vi "TV-HR_Main.vi"(8 "error in":errorcluster) -> (0 "error out":errorcluster)   [LabVIEW 2024]
uses:
  Buttons/Zoom IN.ctl
  Buttons/Zoom Out.ctl
  Buttons/Zoom Inn.ctl
  Buttons/Zoom Fit.ctl
  Buttons/ML Analysis.ctl
  <vilib>/Utility/error.llb/DialogType.ctl
  Controls/RVHR - UI Refs.ctl
  Controls/RVHR - Reporting Settings.ctl
  Controls/RVHR - Local Data.ctl
  Controls/Test Cluster.ctl
  Controls/Excluded Information.ctl
  Controls/Language.ctl
  Controls/Device_Type.ctl
  <vilib>/Utility/miscctls.llb/LVRectTypeDef.ctl
  <vilib>/Utility/miscctls.llb/LVBoundsTypeDef.ctl
  Modules/Error handling/Controls/Error Command.ctl
  Controls/DB FTR Commands.ctl
  <vilib>/Utility/miscctls.llb/LVPoint32TypeDef.ctl
  Controls/Print Command.ctl
  Controls/RVHR - Analysis Mode.ctl
  Controls/Run Listbox Command.ctl
panel:
  in  "Ref Profile":string caption="Ref Profile:"
  in  "Company":string caption="Company:"
  in  "Location":string caption="Location:"
  in  "Operator":string caption="Operator:"
  in  "Notes":string caption="Notes:"
  in  "Date":string caption="Date:"
  in  "Run End":dbl caption="Run End:" format="%.3f km"
  in  "Run Start":dbl caption="Run Start:" format="%.3f km"
  out "new picture":picture
  out "EN Sub-Title":string caption="EN13231-2/EN13231-3"
  out "Sub-Title":string caption="RV-HR Report"
  out "Title":string caption="Rail Vision - HR"
  out "ML Analysis":T1
  in  "All?":bool
  in  "Run Selection Listbox":i32(listbox)
  in  "Feature Type:":u16(ring) items=["Clip", "Crack", "Add New..."]
  in  "Run Distance":dbl(slide) caption="Distance (km)" min=11.015 max=11.025 step=0.002 scale=11.015..11.025
  out "Running?":bool
  in  "Zoom Toolbar L":T5
  out "Rail Preview":picture
  in  "Zoom Window":T6
  out "Image Preview":picture
  in  "Previous?":bool
  in  "Next?":bool
  out "Page":string
  out "Left Rail":string
  out "Image":picture
  # "Left"
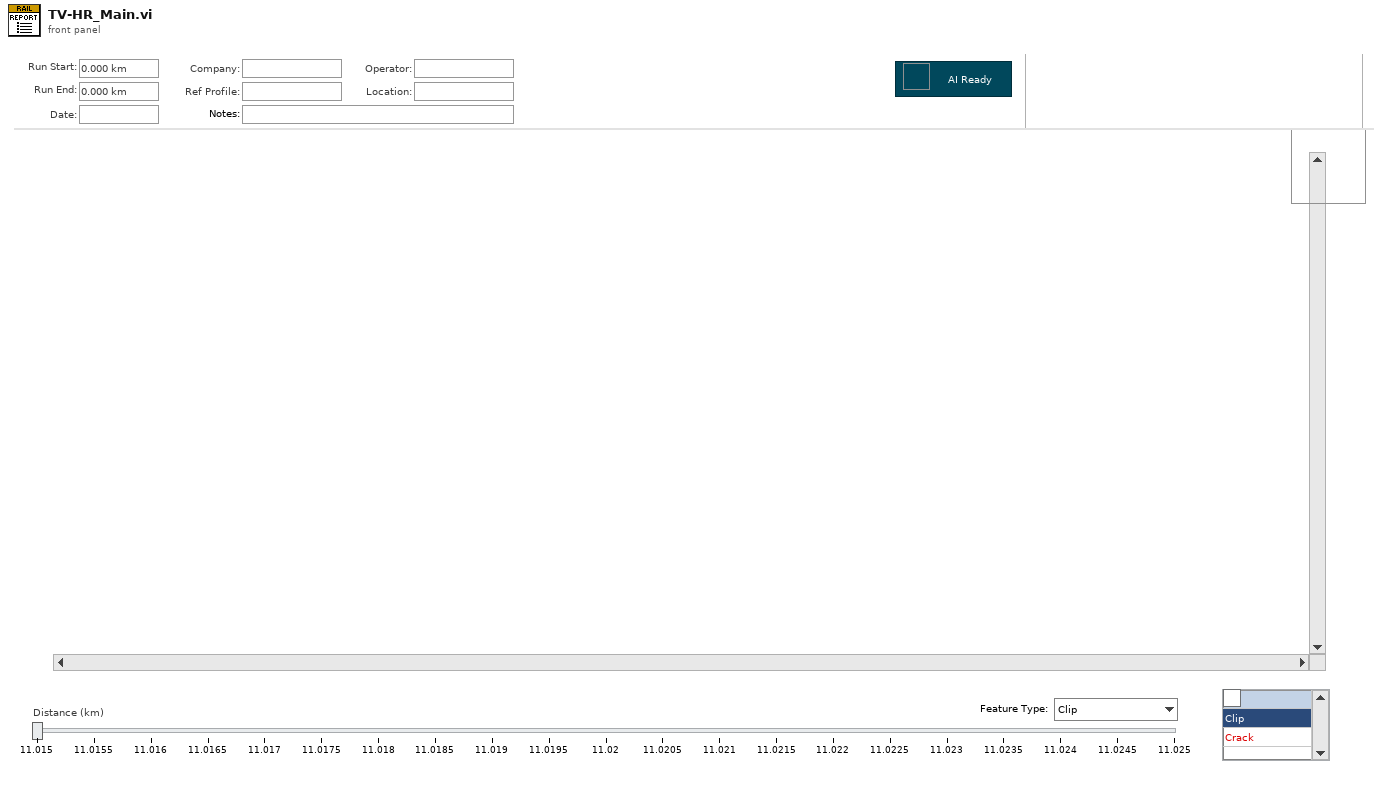
[diagram p1: front panel]
types:
  T1 = typedef "ML Analysis.ctl" = bool
  T2 = typedef "Zoom Out.ctl" = bool
  T3 = typedef "Zoom Inn.ctl" = bool
  T4 = typedef "Zoom Fit.ctl" = bool
  T5 = cluster{"Zoom Out":T2, "Zoom In":T3, "Zoom Fit":T4}
  T6 = typedef "Zoom IN.ctl" = bool
  T7 = typedef "DialogType.ctl" = u16
  T8 = typedef "RVHR - UI Refs.ctl" = cluster{"Title":refnum<vi>, "Sub-Title":refnum<vi>, "EN Sub-Title":refnum<vi>, "Run Start":refnum<vi>, "Run End":refnum<vi>, "Date":refnum<vi>, "Company":refnum<vi>, "Ref Profile":refnum<vi>, "Operator":refnum<vi>, "Location":refnum<vi>, "Notes":refnum<vi>, "Left Rail":refnum<vi>, "Page":refnum<vi>, "Image":refnum<vi>, "Run Distance":refnum<vi>, "Next?":refnum<vi>, "Previous?":refnum<vi>, "Image Preview":refnum<vi>, "Feature Type:":refnum<vi>, "Zoom Toolbar L":refnum<vi>, "Rail Preview":refnum<vi>, "ML Analysis":refnum<vi>, "Running?":refnum<vi>, "All?":refnum<vi>, "Run Selection Listbox":refnum<vi>}
  T9 = typedef "RVHR - Reporting Settings.ctl" = cluster{"Image Distance (m)":dbl}
  T10 = typedef "Error Command.ctl" = enum16{"Initialisation", "Handle", "Close"}
  T11 = enum8{"Enabled", "Disabled", "Disabled and Grayed Out"}
  T12 = typedef "RVHR - Analysis Mode.ctl" = enum16{"Current Images", "Full Run"}
  T13 = enum16{"Get Image", "Get Preview", "Add", "Remove"}
  T14 = cluster{"Label.Text":string, "Mouse Position (Start)":cluster{"X":i32, "Y":i32}}
  T15 = typedef "DB FTR Commands.ctl" = enum16{"Add New", "Get", "Update"}
  T16 = typedef "LVPoint32TypeDef.ctl" = cluster{"Horizontal":i32, "Vertical":i32}
  T17 = typedef "Print Command.ctl" = enum16{"Current Page", "Full Report"}
  T18 = typedef "Run Listbox Command.ctl" = enum16{"Init", "Item Names", "Update", "Update All", "Get Selections", "Clear"}
  T19 = typedef "Language.ctl" = enum16{"English", "Chinese", "German"}
  T20 = typedef "Supervisory Config Cluster.ctl" = cluster{"UI Information":T21, "Test Cluster":T25, "RV-HR Settings Cluster":T26}
  T21 = typedef "UI Init Config Info.ctl" = cluster{"Header Image":path, "Language":T19, "First Run?":bool, "Setup Camera?":bool, "Device Type":T22, "Encoder Type":T23, "Version":T24, "port":i32, "greyscale":bool, "camera index":i32}
  T22 = typedef "Device_Type.ctl" = enum16{"CAT", "Bi-CAT", "YRCA", "RCA", "RV-HR", "TV-HR"}
  T23 = typedef "EncoderType.ctl" = enum16{"Tacho", "Quadrature"}
  T24 = typedef "Software Version.ctl" = enum16{"RailMeasurement_CAT", "RailMeasurement_Master", "RailMeasurement_RCA", "RailMeasurement_CAT-V", "RailMeasurement_RCA-V", "RailMeasurement_RV-HR"}
  T25 = typedef "Test Cluster.ctl" = cluster{"Operator":string, "Description":string, "Line":string, "Start Position":dbl, "Run Length":dbl, "Sensor A Position":dbl, "Rail Side":bool, "Distance Direction":bool, "Path":path, "Sensor B Position":dbl, "Visible Chart Distance":dbl, "Company":string, "Ref Profile":string}
  T26 = typedef "Settings Cluster.ctl" = cluster{"Sensor A Calibration":dbl, "Integrator Time":dbl, "Encoder Spacing":dbl, "Encoder Threshold":dbl, "Sampling Distance":T27, "Swap Direction?":bool, "Min Walking Speed":dbl, "Max Walking Speed":dbl, "Distance Format":T28, "Sensor B Calibration":dbl, "Tacho Pulses/Rev":dbl, "Wheel Diameter":dbl, "Max Short Roughness":dbl, "Max Long Roughness":dbl, "Measuring Interval":dbl, "Measuring Length":dbl, "Wavelengths":dbl[], "Device Resolution":T29, "Detect Change in Direction?":bool, "Save Images?":bool, "Image Frequency":T27, "Save Video?":bool, "Image Offset":dbl, "Start Position at 0m?":bool, "Live Corrug Est.?":bool, "Wavelength Corrug":u8, "Distance Corrug":u8, "Update Corrug":u8}
  T27 = typedef "Sampling DIstance.ctl" = u16
  T28 = typedef "Distance Units.ctl" = u16
  T29 = typedef "Device_Resolution.ctl" = u16
  T30 = typedef "RVHR - Local Data.ctl" = cluster{"Main Filtered Data":dbl[][][], "Main Dist Data":dbl[], "Comp Filtered Data":dbl[][][], "Comp Dist Data":dbl[], "Image":u16, "Total Images":u16, "Main Test Cluster":T25, "Main Dates-Times":cluster{"Start Date":string, "Start Time":string, "Finish Time":string}, "Comp Test Cluster":T25, "Comp Dates-Times":cluster{"Start Date":string, "Start Time":string, "Finish Time":string}, "Comp Offset (mm)":i64, "XY Highlight Distance":dbl[], "Left Exc Info":T31[], "Right Exc Info":T31[], "Custom Start-Point":dbl, "UI Start-Distance":dbl, "UI End-Distance":dbl, "Distance Format":u8, "Language":T19, "Vision?":bool, "Left Image Folder":path, "Filename _L":string[], "Image Distances _L":dbl[], "Image Inc (km)":dbl, "Device Type":T22, "Panel Bounds":T32, "Panel Size":T33, "Version":string, "db Filepath":path, "Image Display Scale Factor":dbl}
  T31 = typedef "Excluded Information.ctl" = cluster{"Start Dist":dbl, "End Dist":dbl, "Comments":string}
  T32 = typedef "LVRectTypeDef.ctl" = cluster{"Left":i16, "Top":i16, "Right":i16, "Bottom":i16}
  T33 = typedef "LVBoundsTypeDef.ctl" = cluster{"Width":u32, "Height":u32}
  T34 = typedef "Language Vision Text Cluster.ctl" = cluster{"Home":string, "Test Setup":string, "Run Test":string, "Configure":string, "Hardware Viewer":string, "Review Test":string, "Report":string, "Exit":string, "Device Connected?":string, "Test in Progress?":string, "Simulate?":string, "Device Type 1":string, "Device Type 2":string, "Device Type 3":string, "Device Type 4":string, "Device Type 5":string, "Device Type 6":string, "Device Type 7":string, "Software Version":string, "Support":string, "Operator":string, "Test Description":string, "Line":string, "Test Folder Path":string, "Test Folder Path RCA":string, "Start Position":string, "Sensor Position":string, "Sensor A Position":string, "Sensor B Position":string, "Visible Chart Distance":string, "Rail Side":string, "Rail A Side":string, "Distance Direction":string, "Start":string, "Distance Travelled":string, "Current Position":string, "Stop Test":string, "Pause Test":string, "Displacement":string, "Position":string, "Sensor Calibration":string, "Sensor A Calibration":string, "Sensor B Calibration":string, "Encoder Spacing":string, "Sampling Distance":string, "Tacho Pulses/Rev":string, "Wheel Diameter":string, "Sampling Distances":string[], "Distance Unit":string, "Distance Units":string[], "Swap Direction":string, "Language":string, "Device Resolution":string, "Device Resolutions":string[], "Detect Change in Direction":string, "Save Config":string, "Encoder Data":string, "Sensor Data":string, "Sensor A Data":string, "Sensor B Data":string, "Voltage":string, "Time (m:s)":string, "Unit mm/s/V":string, "Unit mm":string, "Unit km":string, "Unit m":string, "Start Test Message":string, "Stop Test Message":string, "Exit Message":string, "File Exists Message":string, "File Path Invalid Message":string, "Combine Error":string, "Combine Success":string, "Roller Comp Error":string, "Test Folder Path (Live)":string, "Folder Error":string, "Enc Count":string, "Run Start":string, "Run End":string, "Date":string, "Train":string, "Location":string, "Notes":string, "Heading_1":string, "Heading_2":string, "Left Rail":string, "Right Rail":string, "Left Exclusions":string, "Right Exclusions":string, "Settings":string, "Wavelength Ranges":string, "Y-Axis Limits":string, "Exc Limits":string, "Other Settings":string, "Distance/Page":string, "Distance/Pages":string[], "Gridlines":string, "Report Tolerance":string, "Manual Cut":string, "Plot Colour":string, "Plot Colours":string[], "EN Standard":string, "RiL Standard":string, "Custom Standard":string, "Resolution":string, "Resolutions":string[], "Exceedence Header":string, "Distance (km)":string, "Left (%)":string, "Right (%)":string, "Page":string, "Align":string, "Main":string, "Comparison":string, "Offset":string, "From":string, "To":string, "Of":string, "File":string, "Load New":string, "Load Comparison":string, "Discard Comparison":string, "Print Current Page":string, "Print All Pages":string, "Print Exceedence Report":string, "Plot Main":string, "No Comparison Data to Align":string, "Run Load Error":string, "Report Load Error":string, "Cut":string, "Remove":string, "Config Settings Unsaved":string, "Acquisition Paused":string, "Please Select One Option Below":string, "RCA is Now Stationary":string, "Reporting Setting":string, "Main Abbreviated":string, "Comparison Abbreviated":string, "Exceedence Abbreviated":string, "Align Comparison":string, "Rail Corrugation Analyser Reporting":string, "Show Exc. % in Graph":string, "Evaluate Sections <100m":string, "Evaluate Sections <0.062mile":string, "Section Too Short for Evaluation":string, "Language Change Prompt":string, "Show All":string, "Sections_km":string, "Sections_mi":string, "Vision":string, "Vision Report":string, "Vision Display":string, "Vision Displays":string[], "Save Images":string, "Image Frequency":string, "Section":string, "Brightness":string, "Contrast":string, "Shadow":string, "Sharpened":string, "Apply to all Images":string, "Reset":string, "Are you sure":string, "Image Processing":string, "Save Video":string, "Image Offset":string, "Camera Mode":string, "Camera Modes":string[], "Copy Page":string, "Copy Graphs":string, "Camera Mode Change Prompt":string, "Camera_1 Missing":string, "Camera_2 Missing":string, "Cameras Missing":string, "Camera Setup":string, "Camera_1 Connection Error":string, "Camera_2 Connection Error":string, "Cameras Connection Error":string, "No GPS":string, "No Signal":string, "Camera_1 Connected":string, "Camera_1 Not Connected":string, "Camera_2 Connected":string, "Camera_2 Not Connected":string, "Start Position at 0m?":string, "Continue":string, "New Test, Same Direction":string, "New Test, Opposite Direction":string, "Stop and Save":string, "Live Corrug Estimate":string, "Wavelength Corrug":string, "Distance Corrug ":string, "Update Corrug":string, "Company":string, "Ref Profile ":string, "Company_Report":string, "Ref Profile_Report":string, "Heading_1_RVHR":string, "Heading_2_RVHR":string, "Remove Feature":string, "Feature Type":string, "Feature Types":string[], "AI Not Ready":string}
  T35 = typedef "Vision - Local Data.ctl" = cluster{"Main Filtered Data":dbl[][][], "Main Dist Data":dbl[], "Comp Filtered Data":dbl[][][], "Comp Dist Data":dbl[], "Page":u8, "Total Pages":u8, "Main Test Cluster":T25, "Main Dates-Times":cluster{"Start Date":string, "Start Time":string, "Finish Time":string}, "Comp Test Cluster":T25, "Comp Dates-Times":cluster{"Start Date":string, "Start Time":string, "Finish Time":string}, "Comp Offset (mm)":i64, "XY Highlight Distance":dbl[], "Left Exc Info":T31[], "Right Exc Info":T31[], "Custom Start-Point":dbl, "UI Start-Distance":dbl, "UI End-Distance":dbl, "Distance Format":u8, "Language":T19, "Vision?":bool, "Image Folder":path, "Filename _L":string[], "Filename _R":string[], "Image Distances _L":dbl[], "Image Distances _R":dbl[], "Image Inc (km)":dbl, "Device Type":T22, "Panel Bounds":T32, "Panel Size":T33, "Vision Settings":T36}
  T36 = typedef "Vision - Reporting Settings.ctl" = cluster{"Show All?":bool, "Dist/Page":T37, "Sections":T38[]}
  T37 = typedef "Vision - Dist Per Page.ctl" = u16
  T38 = typedef "Vision - Section.ctl" = cluster{"From":dbl, "To":dbl, "Discard":T39}
  T39 = typedef "Bin.ctl" = bool
  T40 = typedef "imagedata.ctl" = cluster{"image type":i32, "image depth":i32, "image":u8[], "mask":u8[], "colors":u32[], "Rectangle":cluster{"left":i16, "top":i16, "right":i16, "bottom":i16}}
  T41 = typedef "Local Data.ctl" = cluster{"Main Filtered Data":dbl[][][], "Main Dist Data":dbl[], "Comp Filtered Data":dbl[][][], "Comp Dist Data":dbl[], "Page":u8, "Total Pages":u8, "Main Test Cluster":T25, "Main Dates-Times":cluster{"Start Date":string, "Start Time":string, "Finish Time":string}, "Comp Test Cluster":T25, "Comp Dates-Times":cluster{"Start Date":string, "Start Time":string, "Finish Time":string}, "Comp Offset (mm)":i64, "XY Highlight Distance":dbl[], "Left Exc Info":T31[], "Right Exc Info":T31[], "Custom Start-Point":dbl, "UI Start-Distance":dbl, "UI End-Distance":dbl, "Distance Format":u8, "Language":T19, "Main Sampling Distance (mm)":dbl, "Comp Sampling Distance (mm)":dbl}
  T42 = typedef "eventvkey.ctl" = enum16{"ASCII", "Enter", "Return", "Shift", "Ctrl", "Alt", "Cmd", "Opt", "Caps", "NumLock", "Clear", "Break", "Up", "Down", "Left", "Right", "Insert", "Delete", "Home", "End", "PageUp", "PageDown", "Escape", "Help", "Pause", "ScrollLock", "F1", "F2", "F3", "F4", "F5", "F6", "F7", "F8", "F9", "F10", "F11", "F12", "F13", "F14", "F15", "F16", "F17", "F18", "F19", "F20", "F21", "F22", "F23", "F24", "Play", "VolumeUp", "VolumeDown", "Mute", "Two Byte Char"}
  T43 = typedef "LVMouseTypeDef.ctl" = cluster{"Mouse Position":cluster{"X":i32, "Y":i32}, "Mouse Modifiers":cluster{"Button Down":bool, "Shift Mod":bool, "Menu Mod":bool, "Option Mod":bool}}
  T44 = cluster{"Label.Text":string, "Mouse Position":cluster{"X":i32, "Y":i32}}
  T45 = enum32{"invalid app kind", "Development System", "Run Time System", "Student Edition", "Embedded LabVIEW", "Evaluation", "Custom"}
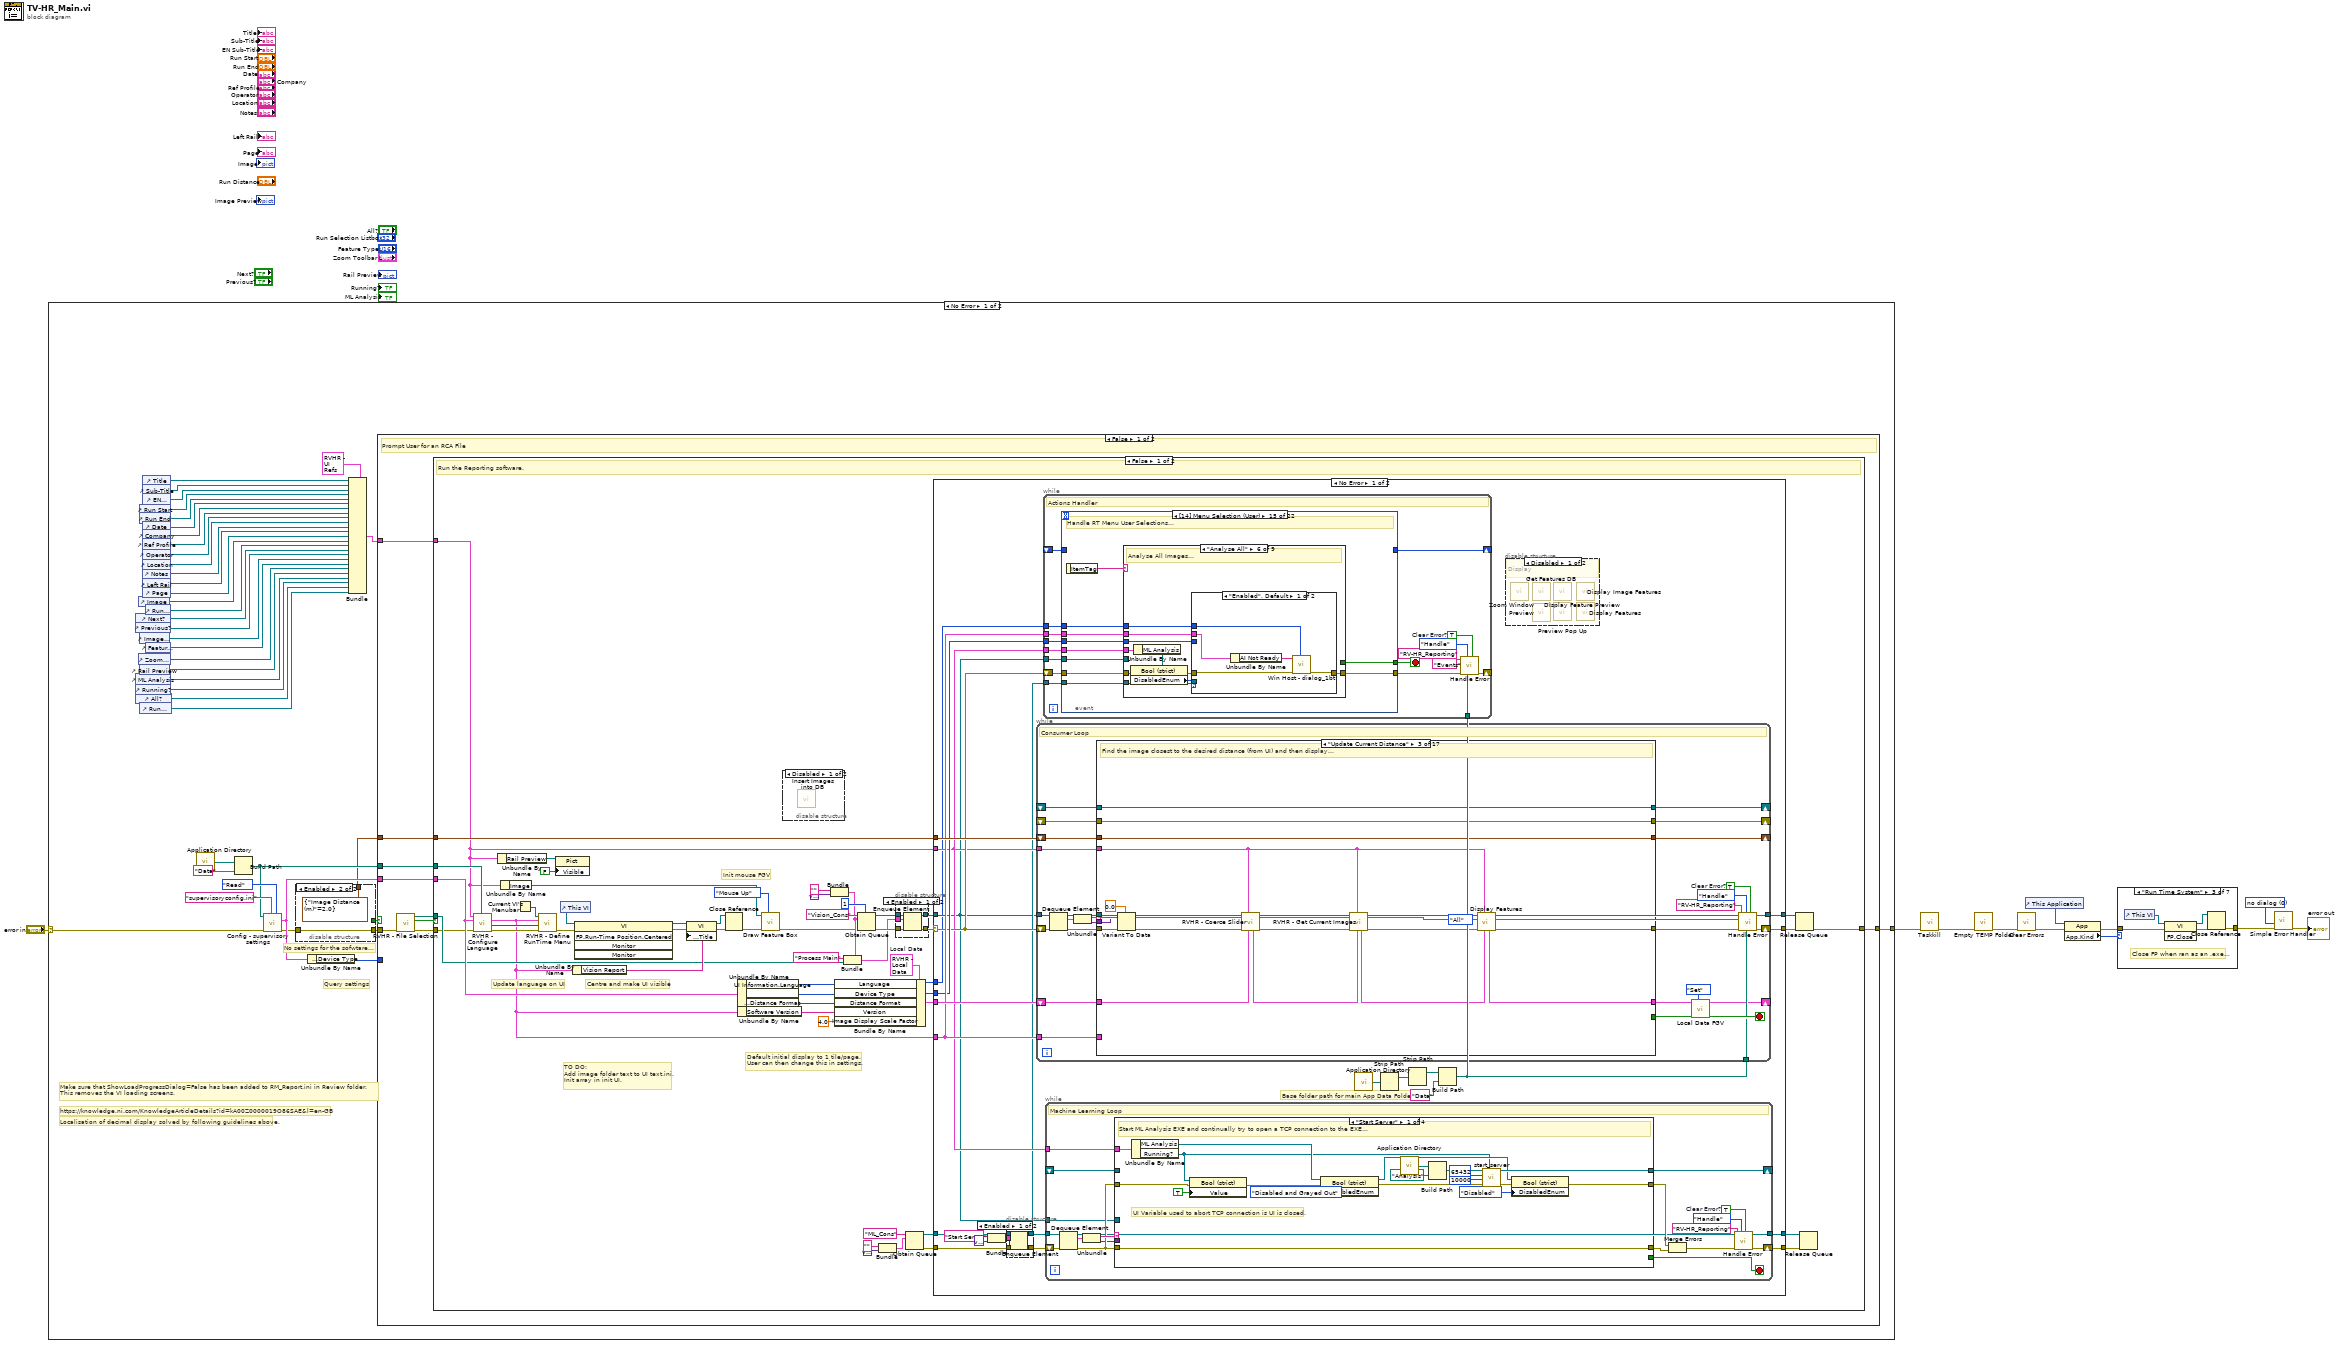
[diagram p0: block diagram]
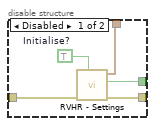
[diagram p2: hidden frame]
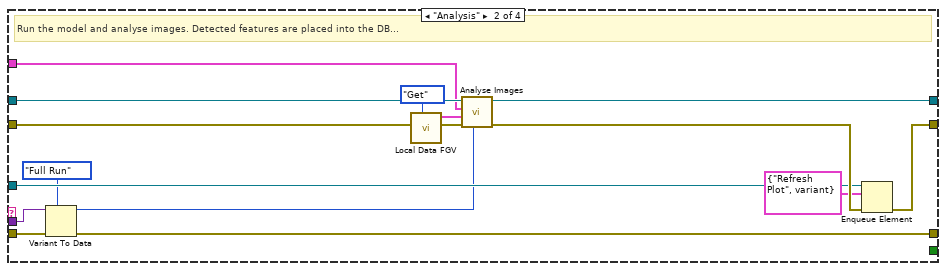
[diagram p6: hidden frame]
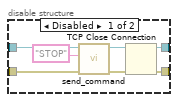
[diagram p8: hidden frame]
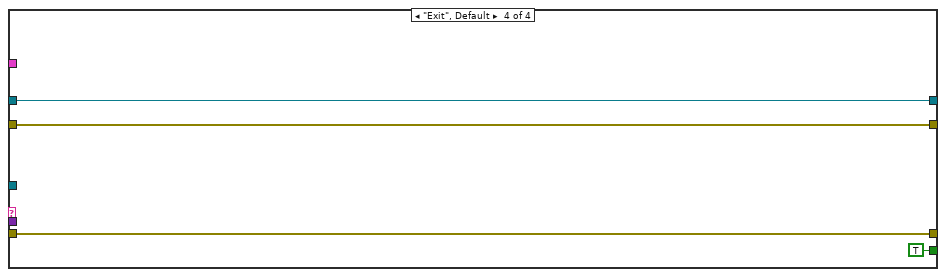
[diagram p9: hidden frame]
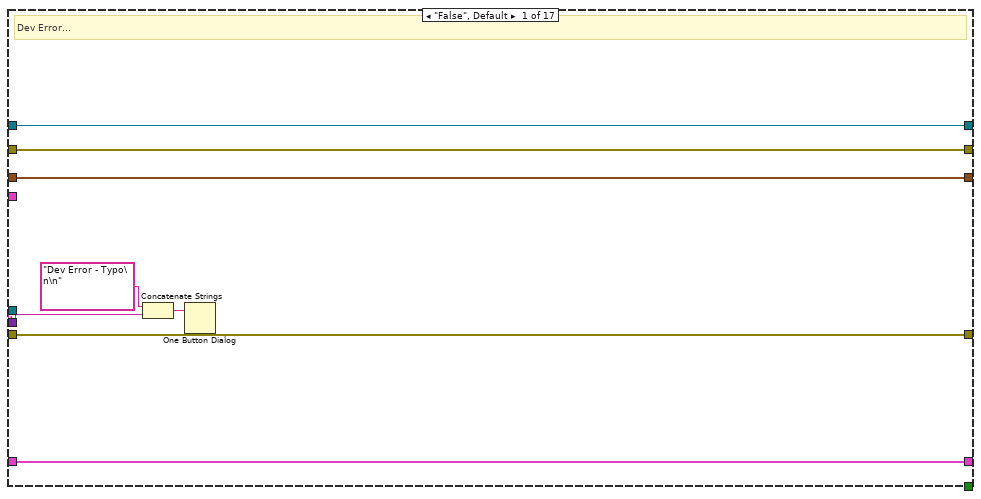
[diagram p11: hidden frame]
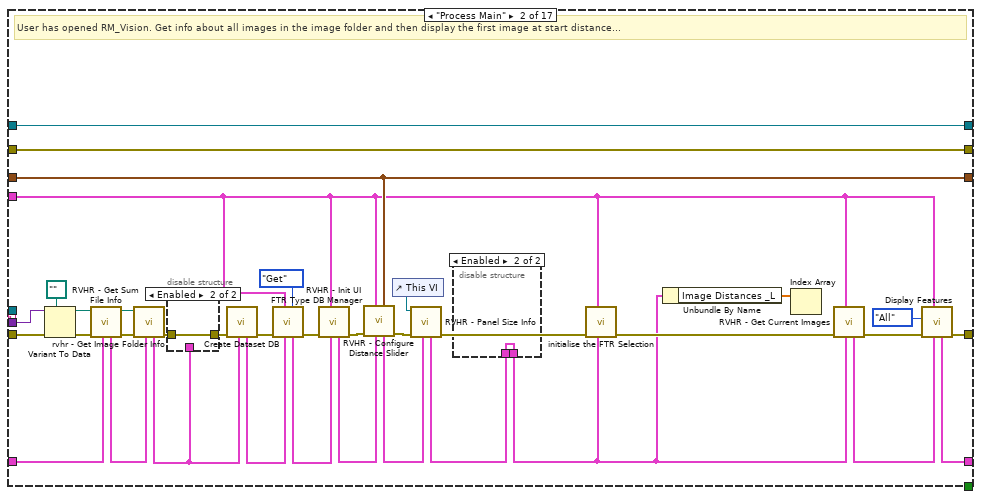
[diagram p12: hidden frame]
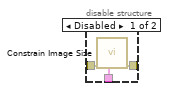
[diagram p13: hidden frame]
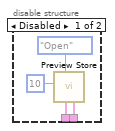
[diagram p14: hidden frame]
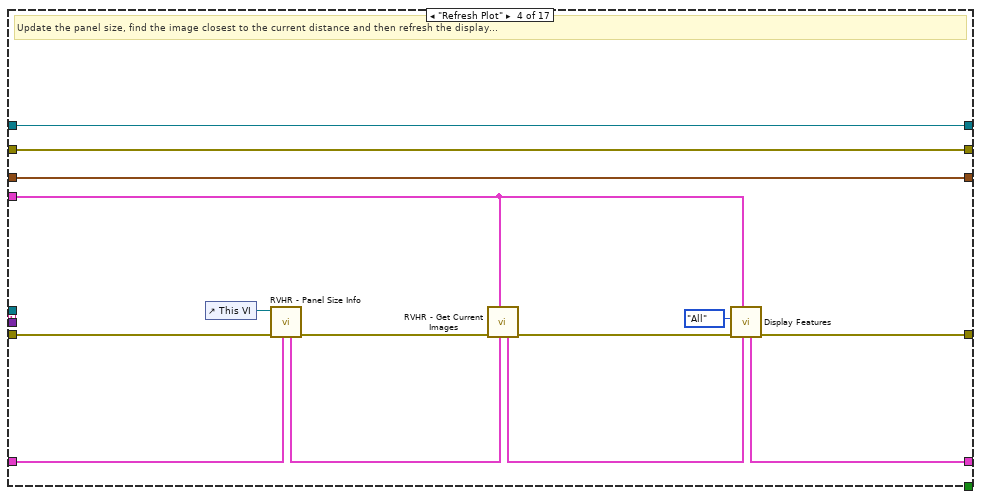
[diagram p15: hidden frame]
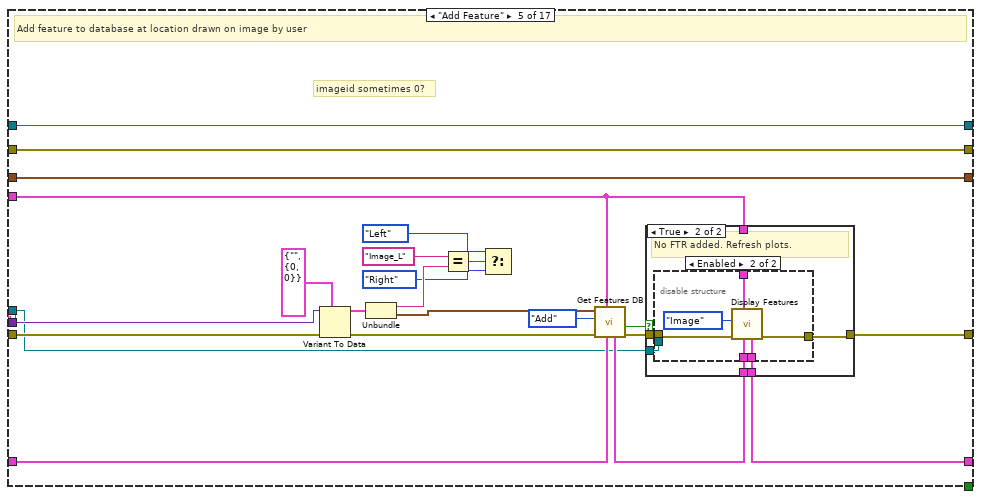
[diagram p16: hidden frame]
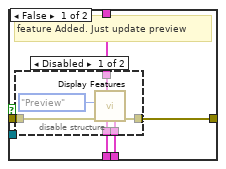
[diagram p17: hidden frame]
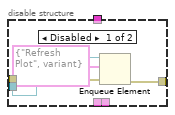
[diagram p19: hidden frame]
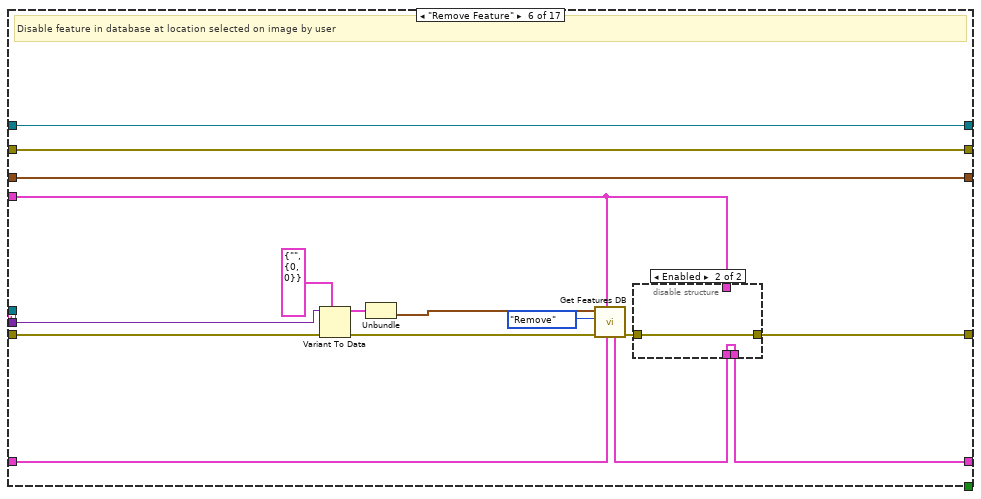
[diagram p20: hidden frame]
diagram:
  w8 = T7 0 items=["no dialog", "OK message", "continue or stop message", "OK message + warnings", "continue/stop + warnings"] ("type of dialog (OK msg:1)")
  n1 = case shown="No Error" "error in" {
    selector: "error in" -> [w18 w1098]
    tunnel: [w42 w1098] -> w5
    frame No Error {
      # "No settings for the sofwtare..."
      # "Make sure that ShowLoadProgressDialog=False has been added to RM_Report.ini in Review folder.\nThis removes the VI loading screens."
      # "Localisation of decimal display solved by following guidelines above."
      # "https://knowledge.ni.com/KnowledgeArticleDetails?id=kA00Z0000019O86SAE&l=en-GB"
      # "Query settings"
      n2 = control-ref of="Next?"() -> (w39:refnum<vi>)
      n3 = control-ref of="Previous?"() -> (w38:refnum<vi>)
      n4 = control-ref of="ML Analysis"() -> (w17:refnum<vi>)
      n5 = control-ref of="Running?"() -> (w16:refnum<vi>)
      n6 = control-ref of="All?"() -> (w14:refnum<vi>)
      n7 = control-ref of="Image"() -> (w19:refnum<vi>)
      n8 = control-ref of="Zoom Toolbar L"() -> (w20:refnum<vi>)
      n9 = control-ref of="Image Preview"() -> (w23:refnum<vi>)
      n10 = control-ref of="Rail Preview"() -> (w21:refnum<vi>)
      n11 = control-ref of="Run Selection Listbox"() -> (w13:refnum<vi>)
      n12 = control-ref of="Run Start"() -> (w31:refnum<vi>)
      n13 = control-ref of="Run End"() -> (w30:refnum<vi>)
      n14 = control-ref of="Title"() -> (w51:refnum<vi>)
      n15 = control-ref of="Sub-Title"() -> (w50:refnum<vi>)
      n16 = control-ref of="EN Sub-Title"() -> (w41:refnum<vi>)
      n17 = control-ref of="Date"() -> (w29:refnum<vi>)
      n18 = control-ref of="Company"() -> (w28:refnum<vi>)
      n19 = control-ref of="Ref Profile"() -> (w27:refnum<vi>)
      n20 = control-ref of="Operator"() -> (w26:refnum<vi>)
      n21 = control-ref of="Location"() -> (w25:refnum<vi>)
      n22 = control-ref of="Notes"() -> (w24:refnum<vi>)
      n23 = control-ref of="Left Rail"() -> (w49:refnum<vi>)
      n24 = control-ref of="Page"() -> (w44:refnum<vi>)
      n25 = control-ref of="Run Distance"() -> (w40:refnum<vi>)
      n26 = control-ref of="Feature Type:"() -> (w22:refnum<vi>)
      n27 = call <vilib>:"Application Directory.vi"() -> ("Application Directory"=w15:path)
      n28 = Build Path(base path=w15, name or relative path="Data") -> (appended path=w36:path)
      n29 = call "Config - supervisory settings.vi"(".ini Controller"=enum16{"Read", "Write"}."Read", ".ini filename"="supervisoryconfig.ini", "error in (no error)"=w18, "Directory Path"=w36) -> ("error out"=w32:errorcluster, "Supervisory Config Cluster Out"=w45:T20)  [unwired: 5 in, 1 out]
      n30 = disable-structure shown="Enabled" {
        disable-tunnel: [w56 T9 {"Image Distance (m)"=2.0} ("Supervisory Config Cluster In")] -> w35
        disable-tunnel: [w55 w58] -> w34
        disable-tunnel: [w54 _] -> w33
        disable-tunnel: w32 -> [w52 w58]
        frame Disabled {
          w53 = TRUE  # Initialise?
          n31 = call "RVHR - Settings.vi"("Initialise?"=w53, "error in (no error)"=w52) -> ("Error"=w55:errorcluster, "Cancelled?"=w54:bool, "Supervisory Config Cluster In"=w56:T9)  [unwired: 7 in]
        }
        frame Enabled {
        }
      }
      n32 = Unbundle By Name(w45) -> ("UI Information.Device Type"=w46:T22)
      n33 = Bundle(cluster=T8 {"Title"=refnum, "Sub-Title"=refnum, "EN Sub-Title"=refnum, "Run Start"=refnum, "Run End"=refnum, "Date"=refnum, "Company"=refnum, "Ref Profile"=refnum, "Operator"=refnum, "Location"=refnum, "Notes"=refnum, "Left Rail"=refnum, "Page"=refnum, "Image"=refnum, "Run Distance"=refnum, "Next?"=refnum, "Previous?"=refnum, "Image Preview"=refnum, "Feature Type:"=refnum, "Zoom Toolbar L"=refnum, "Rail Preview"=refnum, "ML Analysis"=refnum, "Running?"=refnum, "All?"=refnum, "Run Selection Listbox"=refnum} ("output cluster"), "Title"=w51, "Sub-Title"=w50, "EN Sub-Title"=w41, "Run Start"=w31, "Run End"=w30, "Date"=w29, "Company"=w28, "Ref Profile"=w27, "Operator"=w26, "Location"=w25, "Notes"=w24, "Left Rail"=w49, "Page"=w44, "Image"=w19, "Run Distance"=w40, "Next?"=w39, "Previous?"=w38, "Image Preview"=w23, "Feature Type:"=w22, "Zoom Toolbar L"=w20, "Rail Preview"=w21, "ML Analysis"=w17, "Running?"=w16, "All?"=w14, "Run Selection Listbox"=w13) -> (w43:T8)
      n34 = case shown="False" w33 {
        tunnel: w36 -> [w67 _]
        tunnel: w34 -> [w62 w1096]
        tunnel: w46 -> [_ _]
        tunnel: w45 -> [w66 _]
        tunnel: w43 -> [w65 _]
        tunnel: w35 -> [w64 _]
        tunnel: [w63 w1096] -> w42
        frame False {
          # "Prompt User for an RCA File"
          n35 = call "RVHR - File Selection.vi"("error in"=w62) -> ("error out"=w61:errorcluster, "cancelled?"=w60:bool, "RVHR path"=w59:path)  [unwired: 8 in]
          n36 = case shown="False" w60 {
            tunnel: w61 -> [w82 w1095]
            tunnel: w59 -> [w89 _]
            tunnel: w65 -> [w73 _]
            tunnel: w67 -> [w119 _]
            tunnel: w66 -> [w91 _]
            tunnel: w64 -> [w102 _]
            tunnel: [w104 w1094] -> w63
            frame False {
              w105 = T30 {"Main Filtered Data"=[[[0.0]]], "Main Dist Data"=[], "Comp Filtered Data"=[[[0.0]]], "Comp Dist Data"=[], "Image"=0, "Total Images"=0, "Main Test Cluster"={"Operator"="", "Description"="", "Line"="", "Start Position"=0.0, "Run Length"=0.0, "Sensor A Position"=0.0, "Rail Side"=FALSE, "Distance Direction"=FALSE, "Path"=path "", "Sensor B Position"=0.0, "Visible Chart Distance"=0.0, "Company"="", "Ref Profile"=""}, "Main Dates-Times"={"Start Date"="", "Start Time"="", "Finish Time"=""}, "Comp Test Cluster"={"Operator"="", "Description"="", "Line"="", "Start Position"=0.0, "Run Length"=0.0, "Sensor A Position"=0.0, "Rail Side"=FALSE, "Distance Direction"=FALSE, "Path"=path "", "Sensor B Position"=0.0, "Visible Chart Distance"=0.0, "Company"="", "Ref Profile"=""}, "Comp Dates-Times"={"Start Date"="", "Start Time"="", "Finish Time"=""}, "Comp Offset (mm)"=0, "XY Highlight Distance"=[], "Left Exc Info"=[], "Right Exc Info"=[], "Custom Start-Point"=0.0, "UI Start-Distance"=0.0, "UI End-Distance"=0.0, "Distance Format"=0, "Language"=enum."English", "Vision?"=FALSE, "Left Image Folder"=path "", "Filename _L"=[], "Image Distances _L"=[], "Image Inc (km)"=0.0, "Device Type"=enum."CAT", "Panel Bounds"={"Left"=0, "Top"=0, "Right"=0, "Bottom"=0}, "Panel Size"={"Width"=0, "Height"=0}, "Version"="", "db Filepath"=path "", "Image Display Scale Factor"=0.0}  # Local Data
              # "Init mouse FGV"
              # "Default initial display to 1 tile/page.\nUser can then change this in settings."
              # "TO DO:\nAdd image folder text to UI text.ini.\nInit array in init UI."
              # "Update language on UI"
              # "Centre and make UI visible"
              # "Run the Reporting software."
              n37 = call "RVHR - Configure Language.vi"("Directory Path"=w119, "error in (no error)"=w82, "Supervisory Config Cluster Out"=w91, "UI References"=w73) -> ("error out"=w101:errorcluster, "UI Information.Language"=w99:T19, "Language Config Cluster Out"=w70:T34)  [unwired: 4 in, 1 out]
              n38 = Unbundle By Name(w73) -> ("Rail Preview"=w86:refnum<vi>)
              n39 = Unbundle By Name(w73) -> ("Image"=w72:refnum<vi>)
              n40 = Current VI's Menubar() -> (w100:refnum<k9>)
              n41 = call "RVHR - Define RunTime Menu.vi"("error in (no error)"=w101, "Language"=w99, "Language Config Cluster Out"=w70, "Menu in"=w100) -> ("error out"=w98:errorcluster)  [unwired: 7 in]
              n42 = property class="Pict"(reference=w86, "Visible"=FALSE) -> ()  [unwired: 1 in, 2 out]
              n43 = control-ref of="This VI"() -> (w118:refnum<vi>)
              n44 = Unbundle By Name(w70) -> ("Vision Report"=w93:string)
              n45 = invoke class="VI" method="FP.Run-Time Position.Centered"(reference=w118, error in=w98) -> (reference out=w94:refnum<vi>, error out=w95:errorcluster)  [unwired: 3 in, 3 out]
              n46 = property class="VI"(reference=w94, error in=w95, "Front Panel.Title"=w93) -> (reference out=w97:refnum<vi>, error out=w96:errorcluster)
              n47 = Close Reference(reference=w97, error in (no error)=w96) -> (error out=w84:errorcluster)
              n48 = Unbundle By Name(w91) -> ("UI Information.Language"=w69:T19, "UI Information.Device Type"=w90:T22, "RV-HR Settings Cluster.Distance Format"=w92:T28)
              n49 = Unbundle By Name(w70) -> ("Software Version"=w71:string)
              n50 = call "Draw Feature Box.vi"("Action"=enum16{"Mouse Move", "Mouse Down", "Mouse Up"}."Mouse Up", "error in (no error)"=w84, "CtlRef"=w72) -> ("error out"=w83:errorcluster)  [unwired: 6 in, 2 out]
              n51 = disable-structure shown="Disabled" {
                frame Disabled {
                  n52 = call "Insert Images into DB.vi"() -> ()  [unwired: 12 in]
                }
                frame Enabled {
                }
              }
              n53 = Bundle("Command"="", "Data"=variant) -> (w113:cluster{"Command":string, "Data":variant})  [unwired: 1 in]
              n54 = Bundle By Name(cluster=w105, "Language"=w69, "Device Type"=w90, "Distance Format"=w92, "Version"=w71, "Image Display Scale Factor"=4.0) -> (w103:T30)
              n55 = Bundle(cluster=w113, "Command"="Process Main", "Data"=w89) -> (w111:cluster{"Command":string, "Data":variant})
              n56 = Obtain Queue(max queue size (-1, unlimited)=1, name (unnamed)="Vision_Cons", element data type=w113, error in (no error)=w83) -> (queue out=w110:refnum<queue>, error out=w115:errorcluster)  [unwired: 1 in, 1 out]
              n57 = Bundle("Command"="", "Data"=variant) -> (w80:cluster{"Command":string, "Data":variant})  [unwired: 1 in]
              n58 = disable-structure shown="Enabled" {
                disable-tunnel: w115 -> [w124 w125]
                disable-tunnel: w111 -> [w123 _]
                disable-tunnel: w110 -> [w122 w126]
                disable-tunnel: [w121 w126] -> w109
                disable-tunnel: [w120 w125] -> w85
                frame Enabled {
                  n59 = Enqueue Element(queue=w122, element=w123, error in (no error)=w124) -> (queue out=w121:refnum<queue>, error out=w120:errorcluster)  [unwired: 1 in, 1 out]
                }
                frame Disabled {
                }
              }
              n60 = Obtain Queue(name (unnamed)="ML_Cons", element data type=w80) -> (queue out=w77:refnum<queue>, error out=w76:errorcluster)  [unwired: 3 in, 1 out]
              n61 = case shown="No Error" w85 {
                selector: w85 -> [w140 w1090]
                tunnel: w109 -> [w128 w1091]
                tunnel: [w150 w1091] -> w108
                tunnel: [w149 errorcluster {"status"=FALSE, "code"=0, "source"=""} ("error IO")] -> w107
                tunnel: w102 -> [w148 _]
                tunnel: w73 -> [w139 _]
                tunnel: w103 -> [w147 w1085]
                tunnel: w70 -> [w142 w1087]
                tunnel: w90 -> [w141 _]
                tunnel: w77 -> [w130 w1083]
                tunnel: w76 -> [w132 w1082]
                tunnel: [w137 w1082] -> w75
                tunnel: [w136 w1083] -> w74
                tunnel: w69 -> [w127 _]
                frame No Error {
                  # "Base folder path for main App Data Folder"
                  n62 = Bundle("Command"="Start Server", "Data"=variant) -> (w133:cluster{"Command":string, "Data":variant})  [unwired: 1 in]
                  n63 = disable-structure shown="Enabled" {
                    disable-tunnel: w133 -> [w155 _]
                    disable-tunnel: w132 -> [w154 w156]
                    disable-tunnel: [w153 w156] -> w131
                    disable-tunnel: w130 -> [w152 w157]
                    disable-tunnel: [w151 w157] -> w129
                    frame Enabled {
                      n64 = Enqueue Element(queue=w152, element=w155, error in (no error)=w154) -> (queue out=w151:refnum<queue>, error out=w153:errorcluster)  [unwired: 1 in, 1 out]
                    }
                    frame Disabled {
                    }
                  }
                  n65 = while {
                    shift-right: [w174] -> _
                    shift-left: _ -> [w173]
                    tunnel: w139 -> [w172]
                    tunnel: w129 -> [w171]
                    shift-right: [w162] -> w137
                    shift-left: w131 -> [w170]
                    tunnel: [w161] -> w136
                    tunnel: w128 -> [w159]
                    stop <- w160 stop-if-true
                    w166 = TRUE  # Clear Error?
                    # "Machine Learning Loop"
                    n66 = Dequeue Element(queue=w171, error in (no error)=w170) -> (queue out=w161:refnum<queue>, element=w176:cluster{"Command":string, "Data":variant}, error out=w167:errorcluster)  [unwired: 1 in, 1 out]
                    n67 = Unbundle(w176) -> ("Command"=w175:string, "Data"=w158:variant)
                    n68 = case shown="\"Start Server\"" w175 {
                      tunnel: [w185 w204 w215 w227] -> w169
                      tunnel: w167 -> [w181 w207 w212 w227]
                      tunnel: [w191 w210 w214 w228] -> w174
                      tunnel: w173 -> [_ w209 w213 w228]
                      tunnel: w172 -> [w189 w206 _ _]
                      tunnel: w167 -> [w190 w208 w211 w226]
                      tunnel: [w190 w201 w211 w226] -> w168
                      tunnel: [_ _ _ TRUE] -> w160
                      tunnel: w159 -> [_ w203 _ _]
                      tunnel: w158 -> [_ w200 _ _]
                      frame "Start Server" {
                        # "UI Variable used to abort TCP connection is UI is closed."
                        # "Start ML Analysis EXE and continually try to open a TCP connection to the EXE..."
                        n69 = Unbundle By Name(w189) -> ("ML Analysis"=w188:refnum<vi>, "Running?"=w178:refnum<vi>)
                        n70 = property class="Bool (strict)"(reference=w178, error in=w181, "Value"=T1 TRUE) -> (error out=w180:errorcluster)  [unwired: 1 out]
                        n71 = property class="Bool (strict)"(reference=w188, error in=w180, "DisabledEnum"=T11."Disabled and Grayed Out" ("Disabled")) -> (reference out=w182:refnum<vi>, error out=w187:errorcluster)
                        n72 = call <vilib>:"Application Directory.vi"() -> ("Application Directory"=w192:path)
                        n73 = Build Path(base path=w192, name or relative path=path "Analysis") -> (appended path=w195:path)
                        n74 = call "start_server.vi"("Running?"=w178, "error in (no error)"=w187, "Max. connection attempts"=10000, "port"=u16 65432, "exe directory"=w195) -> ("error out"=w186:errorcluster, "connection ID"=w191:refnum<k5>)  [unwired: 5 in]
                        n75 = property class="Bool (strict)"(reference=w182, error in=w186, "DisabledEnum"=T11."Disabled" ("Disabled")) -> (error out=w185:errorcluster)  [unwired: 1 out]
                      }
                      frame "Analysis" {
                        # "Run the model and analyse images. Detected features are placed into the DB..."
                        n76 = Variant To Data(error in=w208, type=RVHR_-_Analysis_Mode."Full Run" ("Analysis Mode"), Variant=w200) -> (data=w198:T12, error out=w201:errorcluster)
                        n77 = call "Local Data FGV.vi"("Action"=enum16{"Set", "Get"}."Get") -> ("Local Data 2"=w196:T30)  [unwired: 10 in]
                        n78 = call "Analyse Images.vi"("Analysis Mode"=w198, "error in (no error)"=w207, "Local Data in"=w196, "UI Refs"=w206, "TCP Network Connection in"=w209) -> ("error out"=w205:errorcluster, "TCP Network Connection out"=w210:refnum<k5>)  [unwired: 5 in]
                        n79 = Enqueue Element(queue=w203, element=cluster{"Command":string, "Data":variant} {"Command"="Refresh Plot", "Data"=variant}, error in (no error)=w205) -> (error out=w204:errorcluster)  [unwired: 1 in, 2 out]
                      }
                      frame "Stop Server" {
                        n80 = disable-structure shown="Enabled" {
                          disable-tunnel: [w219 w223] -> w215
                          disable-tunnel: [w218 w224] -> w214
                          disable-tunnel: w213 -> [w217 w224]
                          disable-tunnel: w212 -> [w216 w223]
                          frame Disabled {
                            n81 = call "send_command.vi"("error in (no error)"=w216, "command"="STOP", "connection ID"=w217) -> ("error out"=w221:errorcluster, "connection ID out"=w222:refnum<k5>)  [unwired: 6 in, 1 out]
                            n82 = TCP Close Connection(connection ID=w222, error in (no error)=w221) -> (connection ID out=w218:refnum<k5>, error out=w219:errorcluster)  [unwired: 1 in]
                          }
                          frame Enabled {
                          }
                        }
                      }
                      frame "Exit", Default {
                      }
                    }
                    n83 = Merge Errors(w169, w168) -> (w163:errorcluster)
                    n84 = call "Handle Error.vi"("Clear Error?"=w166, "Command"=Error_Command."Handle", "error in (no error)"=w163, "Test Name"="RV-HR_Reporting") -> ("error out"=w162:errorcluster)  [unwired: 5 in, 2 out]
                  }
                  n85 = call <vilib>:"Application Directory.vi"() -> ("Application Directory"=w144:path)
                  n86 = Strip Path(path=w144) -> (stripped path=w145:path)  [unwired: 1 out]
                  n87 = Strip Path(path=w145) -> (stripped path=w146:path)  [unwired: 1 out]
                  n88 = Build Path(base path=w146, name or relative path="Data") -> (appended path=w138:path)
                  n89 = while {
                    tunnel: w128 -> [w254]
                    tunnel: [w232] -> w150
                    shift-right: [w244] -> w149
                    shift-left: w140 -> [w253]
                    tunnel: w139 -> [w248]
                    shift-right: [w229] -> _
                    shift-left: w147 -> [w231]
                    shift-right: [w246] -> _
                    shift-left: w148 -> [w247]
                    tunnel: w138 -> [w239]
                    tunnel: w142 -> [w238]
                    shift-right: [w234] -> _
                    shift-left: _ -> [w236]
                    shift-right: [w235] -> _
                    shift-left: _ -> [w237]
                    stop <- w249 stop-if-true
                    w240 = TRUE  # Clear Error?
                    # "Consumer Loop"
                    n90 = Dequeue Element(queue=w254, error in (no error)=w253) -> (queue out=w232:refnum<queue>, element=w252:cluster{"Command":string, "Data":variant}, error out=w250:errorcluster)  [unwired: 1 in, 1 out]
                    n91 = Unbundle(w252) -> ("Command"=w242:string, "Data"=w251:variant)
                    n92 = case shown="\"Update Current Distance\"" w242 {
                      selector: w242 -> [w257 _ _ _ _ _ _ _ _ _ _ _ _ _ _ _ _]
                      tunnel: w251 -> [_ w295 w321 _ w357 w402 _ w424 w448 w483 _ _ _ _ _ _ _]
                      tunnel: w250 -> [w260 w296 w322 w335 w358 w403 w419 w426 w449 w484 w499 w513 w526 w541 w576 w656 w680]
                      tunnel: [w260 w267 w311 w328 w342 w392 w418 w433 w440 w477 w488 w504 w522 w545 w575 w652 w684] -> w245
                      tunnel: [_ _ _ _ _ _ _ _ _ _ _ _ _ _ _ _ TRUE] -> w249
                      tunnel: w248 -> [_ w264 w313 w331 w340 w395 w420 w434 w439 w480 w491 w506 w523 w546 w573 w650 _]
                      tunnel: w247 -> [w261 w284 w323 w337 w360 w405 w422 w436 w452 w485 w494 w508 w517 w544 w577 w649 w681]
                      tunnel: [w262 w280 w310 w327 w341 w393 w416 w431 w437 w475 w489 w503 w525 w547 w574 w655 w682] -> w230
                      tunnel: w231 -> [w262 w293 w316 w334 w359 w404 w417 w432 w437 w476 w497 w509 w524 w542 w574 w655 w683]
                      tunnel: [w261 w284 w323 w337 w360 w405 w422 w436 w452 w485 w494 w508 w518 w544 w577 w649 w681] -> w246
                      tunnel: w238 -> [_ _ _ _ _ _ _ _ _ _ _ _ w516 w543 _ w653 _]
                      tunnel: w237 -> [w256 w277 w309 w326 w344 w391 w415 w430 w451 w474 w487 w501 w515 w540 w572 w648 w679]
                      tunnel: w236 -> [w255 w276 w308 w325 w343 w390 w414 w429 w450 w473 w486 w500 w514 w539 w571 w647 w678]
                      tunnel: [w256 w277 w309 w326 w344 w391 w415 w430 w451 w474 w487 w501 w515 w540 w570 w648 w679] -> w235
                      tunnel: [w255 w276 w308 w325 w343 w390 w414 w429 w450 w473 w486 w500 w514 w539 w569 w647 w678] -> w234
                      tunnel: w232 -> [_ _ _ _ w338 _ _ _ _ _ _ _ _ _ _ _ _]
                      frame "False", Default {
                        # "Dev Error..."
                        n93 = Concatenate Strings("Dev Error - Typo\n\n" ("message"), w257) -> (w259:string)
                        n94 = One Button Dialog(message=w259) -> ()  [unwired: 1 in, 1 out]
                      }
                      frame "Process Main" {
                        # "User has opened RM_Vision. Get info about all images in the image folder and then display the first image at start distance..."
                        n95 = Variant To Data(error in=w296, type=path "" ("Run Path"), Variant=w295) -> (data=w269:path, error out=w294:errorcluster)
                        n96 = call "RVHR - Get Sum File Info.vi"("Local Data in"=w293, "error in (no error)"=w294, ".sum filepath"=w269) -> ("error out"=w287:errorcluster, "Local Data out"=w292:T30)  [unwired: 7 in]
                        n97 = call "rvhr - Get Image Folder Info.vi"("Local Data in"=w292, "error in (no error)"=w287, "selected path"=w269) -> ("error out"=w271:errorcluster, "Local Data out"=w270:T30)  [unwired: 6 in, 1 out]
                        n98 = disable-structure shown="Enabled" {
                          disable-tunnel: w271 -> [w300 w301]
                          disable-tunnel: w270 -> [w299 _]
                          disable-tunnel: [w298 w301] -> w268
                          frame Disabled {
                            n99 = call "Constrain Image Size.vi"("Local Data in"=w299, "error in (no error)"=w300) -> ("error out"=w298:errorcluster)  [unwired: 9 in]
                          }
                          frame Enabled {
                          }
                        }
                        n100 = call "Create Dataset DB.vi"("Local Data in"=w270, "error in (no error)"=w268) -> ("error out"=w283:errorcluster, "Local Data out"=w274:T30)  [unwired: 8 in]
                        n101 = call "FTR Type DB Manager.vi"("Command"=enum16{"Add New", "Get"}."Get", "Local Data in"=w274, "UI Refs"=w264, "error in (no error)"=w283) -> ("error out"=w275:errorcluster, "Local Data out"=w273:T30)  [unwired: 6 in]
                        n102 = call "RVHR - Init UI.vi"("Local Data in"=w273, "UI Refs"=w264, "error in (no error)"=w275) -> ("error out"=w285:errorcluster, "Local Data out"=w286:T30)  [unwired: 7 in]
                        n103 = call "RVHR - Configure Distance Slider.vi"("Settings"=w284, "Local Data in"=w286, "UI Refs"=w264, "error in (no error)"=w285) -> ("error out"=w291:errorcluster, "Local Data out"=w290:T30)  [unwired: 6 in]
                        n104 = control-ref of="This VI"() -> (w289:refnum<vi>)
                        n105 = call "RVHR - Panel Size Info.vi"("Local Data in"=w290, "error in (no error)"=w291, "This VI"=w289) -> ("error out"=w266:errorcluster, "Local Data out"=w278:T30)  [unwired: 7 in]
                        n106 = disable-structure shown="Enabled" {
                          disable-tunnel: w278 -> [w304 w306]
                          disable-tunnel: [w303 w306] -> w263
                          frame Disabled {
                            n107 = call "Preview Store.vi"("Local Data in"=w304, "Action"=enum16{"Open", "Get", "Close"}."Open", "% resolution"=10) -> ("Local Data out"=w303:T30)  [unwired: 7 in, 1 out]
                          }
                          frame Enabled {
                          }
                        }
                        n108 = call "initialise the FTR Selection.vi"("Local Data in"=w263, "UI Refs"=w264, "error in (no error)"=w266) -> ("error out"=w265:errorcluster)  [unwired: 8 in]
                        n109 = Unbundle By Name(w263) -> ("Image Distances _L"=w288:dbl[])
                        n110 = Index Array(array=w288) -> ()  [unwired: 1 in, 1 out]
                        n111 = call "RVHR - Get Current Images.vi"("Local Data in"=w263, "UI Refs"=w264, "error in (no error)"=w265) -> ("error out"=w282:errorcluster, "Local Data out"=w281:T30)  [unwired: 7 in]
                        n112 = call "Display Features.vi"("Local Data in"=w281, "UI References"=w264, "error in (no error)"=w282, "Action"=enum16{"All", "Preview", "Image"}."All") -> ("error out"=w267:errorcluster, "Local Data out"=w280:T30)  [unwired: 6 in]
                      }
                      frame "Update Current Distance" {
                        # "Find the image closest to the desired distance (from UI) and then display..."
                        n113 = Variant To Data(error in=w322, type=0.0, Variant=w321) -> (data=w319:dbl, error out=w318:errorcluster)
                        n114 = call "RVHR - Coerce Slider.vi"("Local Data in"=w316, "UI Refs"=w313, "error in (no error)"=w318, "New Distance"=w319) -> ("error out"=w317:errorcluster, "Local Data out"=w307:T30)  [unwired: 5 in, 1 out]
                        n115 = call "RVHR - Get Current Images.vi"("Local Data in"=w307, "UI Refs"=w313, "error in (no error)"=w317) -> ("error out"=w315:errorcluster, "Local Data out"=w314:T30)  [unwired: 7 in]
                        n116 = call "Display Features.vi"("Local Data in"=w314, "UI References"=w313, "error in (no error)"=w315, "Action"=enum16{"All", "Preview", "Image"}."All") -> ("error out"=w311:errorcluster, "Local Data out"=w310:T30)  [unwired: 6 in]
                      }
                      frame "Refresh Plot" {
                        # "Update the panel size, find the image closest to the current distance and then refresh the display..."
                        n117 = control-ref of="This VI"() -> (w336:refnum<vi>)
                        n118 = call "RVHR - Panel Size Info.vi"("Local Data in"=w334, "error in (no error)"=w335, "This VI"=w336) -> ("error out"=w324:errorcluster, "Local Data out"=w333:T30)  [unwired: 7 in]
                        n119 = call "RVHR - Get Current Images.vi"("Local Data in"=w333, "UI Refs"=w331, "error in (no error)"=w324) -> ("error out"=w332:errorcluster, "Local Data out"=w329:T30)  [unwired: 7 in]
                        n120 = call "Display Features.vi"("Local Data in"=w329, "UI References"=w331, "error in (no error)"=w332, "Action"=enum16{"All", "Preview", "Image"}."All") -> ("error out"=w328:errorcluster, "Local Data out"=w327:T30)  [unwired: 6 in]
                      }
                      frame "Add Feature" {
                        # "imageid sometimes 0?"
                        # "Add feature to database at location drawn on image by user"
                        n121 = Variant To Data(error in=w358, type=T14 {"Label.Text"="", "Mouse Position (Start)"={"X"=0, "Y"=0}} ("output cluster"), Variant=w357) -> (data=w354:T14, error out=w356:errorcluster)
                        n122 = Unbundle(w354) -> ("Label.Text"=w351:string, "Mouse Position (Start)"=w353:cluster{"X":i32, "Y":i32})
                        n123 = Equal?(x="Image_L", y=w351) -> (x = y?=w350:bool)
                        n124 = Select(t=enum16{"Left", "Right"}."Left" ("Side"), s=w350, f=enum16{"Left", "Right"}."Right" ("Side")) -> ()  [unwired: 1 out]
                        n125 = call "Get Features DB.vi"("Local Data in"=w359, "UI References"=w340, "error in (no error)"=w356, "Action"=T13."Add", "Mouse Position (Start)"=w353) -> ("error out"=w346:errorcluster, "Refresh?"=w339:bool, "Local Data out"=w345:T30)  [unwired: 2 in, 2 out]
                        n126 = case shown="True" w339 {
                          tunnel: w346 -> [w365 w379]
                          tunnel: w345 -> [w364 w376]
                          tunnel: [w363 w378] -> w342
                          tunnel: [w362 w375] -> w341
                          tunnel: w340 -> [w361 w374]
                          tunnel: w338 -> [_ w377]
                          frame False {
                            # "feature Added. Just update preview"
                            n127 = disable-structure shown="Disabled" {
                              disable-tunnel: w365 -> [w371 w373]
                              disable-tunnel: w364 -> [w369 w372]
                              disable-tunnel: [w368 w373] -> w363
                              disable-tunnel: [w367 w372] -> w362
                              disable-tunnel: w361 -> [w366 _]
                              frame Disabled {
                                n128 = call "Display Features.vi"("Local Data in"=w369, "UI References"=w366, "error in (no error)"=w371, "Action"=enum16{"All", "Preview", "Image"}."Preview") -> ("error out"=w368:errorcluster, "Local Data out"=w367:T30)  [unwired: 6 in]
                              }
                              frame Enabled {
                              }
                            }
                          }
                          frame True {
                            # "No FTR added. Refresh plots."
                            n129 = disable-structure shown="Enabled" {
                              disable-tunnel: w379 -> [w382 w388]
                              disable-tunnel: [w381 w389] -> w378
                              disable-tunnel: w377 -> [w380 _]
                              disable-tunnel: w376 -> [_ w387]
                              disable-tunnel: [_ w386] -> w375
                              disable-tunnel: w374 -> [_ w385]
                              frame Disabled {
                                n130 = Enqueue Element(queue=w380, element=cluster{"Command":string, "Data":variant} {"Command"="Refresh Plot", "Data"=variant} ("output cluster"), error in (no error)=w382) -> (error out=w381:errorcluster)  [unwired: 1 in, 2 out]
                              }
                              frame Enabled {
                                n131 = call "Display Features.vi"("Local Data in"=w387, "UI References"=w385, "error in (no error)"=w388, "Action"=enum16{"All", "Preview", "Image"}."Image") -> ("error out"=w389:errorcluster, "Local Data out"=w386:T30)  [unwired: 6 in]
                              }
                            }
                          }
                        }
                      }
                      frame "Remove Feature" {
                        # "Disable feature in database at location selected on image by user"
                        n132 = Variant To Data(error in=w403, type=T14 {"Label.Text"="", "Mouse Position (Start)"={"X"=0, "Y"=0}} ("output cluster"), Variant=w402) -> (data=w399:T14, error out=w401:errorcluster)
                        n133 = Unbundle(w399) -> ("Mouse Position (Start)"=w398:cluster{"X":i32, "Y":i32})  [unwired: 1 out]
                        n134 = call "Get Features DB.vi"("Local Data in"=w404, "UI References"=w395, "error in (no error)"=w401, "Action"=T13."Remove", "Mouse Position (Start)"=w398) -> ("error out"=w396:errorcluster, "Local Data out"=w394:T30)  [unwired: 2 in, 3 out]
                        n135 = disable-structure shown="Enabled" {
                          disable-tunnel: w396 -> [w410 w413]
                          disable-tunnel: w395 -> [w409 _]
                          disable-tunnel: w394 -> [w408 w412]
                          disable-tunnel: [w407 w412] -> w393
                          disable-tunnel: [w406 w413] -> w392
                          frame Disabled {
                            n136 = call "Display Features.vi"("Local Data in"=w408, "UI References"=w409, "error in (no error)"=w410, "Action"=enum16{"All", "Preview", "Image"}."Preview") -> ("error out"=w406:errorcluster, "Local Data out"=w407:T30)  [unwired: 6 in]
                          }
                          frame Enabled {
                          }
                        }
                      }
                      frame "Add New feature Type" {
                        n137 = call "FTR Type DB Manager.vi"("Command"=DB_FTR_Commands."Add New", "Local Data in"=w417, "UI Refs"=w420, "error in (no error)"=w419) -> ("error out"=w418:errorcluster, "Local Data out"=w416:T30)  [unwired: 6 in]
                      }
                      frame "Edit Feature" {
                        n138 = Variant To Data(error in=w426, type=T14 {"Label.Text"="", "Mouse Position (Start)"={"X"=0, "Y"=0}} ("output cluster"), Variant=w424) -> (data=w427:T14, error out=w425:errorcluster)
                        n139 = Unbundle(w427) -> ("Mouse Position (Start)"=w423:cluster{"X":i32, "Y":i32})  [unwired: 1 out]
                        n140 = call "FTR Type DB Manager.vi"("Command"=DB_FTR_Commands."Update", "Local Data in"=w432, "UI Refs"=w434, "error in (no error)"=w425, "Mouse Position (Start)"=w423) -> ("error out"=w433:errorcluster, "Local Data out"=w431:T30)  [unwired: 5 in]
                      }
                      frame "Preview Click" {
                        n141 = Variant To Data(error in=w449, type=0.0 ("x/y"), Variant=w448) -> (data=w441:dbl, error out=w442:errorcluster)
                        n142 = Unbundle By Name(w439) -> ("Run Distance"=w446:refnum<vi>)
                        n143 = Unbundle By Name(w437) -> ("Main Test Cluster.Distance Direction"=w438:bool)
                        n144 = case shown="True" w438 {
                          tunnel: [w462 w472] -> w447
                          tunnel: w446 -> [w460 w471]
                          tunnel: [w459 w470] -> w445
                          tunnel: [w455 w468] -> w444
                          tunnel: w442 -> [w454 w467]
                          tunnel: w441 -> [w453 w466]
                          frame False {
                            n145 = property class="Slide (strict)"(reference=w460, error in=w454) -> (reference out=w462:refnum<vi>, error out=w459:errorcluster, "Scale.Maximum"=w461:dbl, "Scale.Minimum"=w456:dbl)
                            n146 = Subtract(x=w461, y=w456) -> (x-y=w458:dbl)
                            n147 = Multiply(x=w453, y=w458) -> (x*y=w457:dbl)
                            n148 = Add(x=w457, y=w456) -> (x+y=w455:dbl)
                          }
                          frame True {
                            n149 = property class="Slide (strict)"(reference=w471, error in=w467) -> (reference out=w472:refnum<vi>, error out=w470:errorcluster, "Scale.Maximum"=w465:dbl, "Scale.Minimum"=w464:dbl)
                            n150 = Subtract(x=w465, y=w464) -> (x-y=w469:dbl)
                            n151 = Multiply(x=w466, y=w469) -> (x*y=w463:dbl)
                            n152 = Subtract(x=w465, y=w463) -> (x-y=w468:dbl)
                          }
                        }
                        n153 = property class="Slide (strict)"(reference=w447, error in=w445, "Val(Sgnl)"=w444) -> (error out=w440:errorcluster)  [unwired: 1 out]
                      }
                      frame "Preview" {
                        n154 = Variant To Data(error in=w484, type=cluster{"Label.Text":string, "Coords":T16} {"Label.Text"="", "Coords"={"Horizontal"=0, "Vertical"=0}} ("output cluster"), Variant=w483) -> (data=w481:cluster{"Label.Text":string, "Coords":T16}, error out=w478:errorcluster)
                        n155 = Unbundle(w481) -> ("Coords"=w479:T16)  [unwired: 1 out]
                        n156 = call "Preview.vi"("Local Data"=w476, "UI Refs"=w480, "error in (no error)"=w478, "Coords"=w479) -> ("error out"=w477:errorcluster, "Local Data out"=w475:T30)  [unwired: 6 in]
                      }
                      frame "Next Page" {
                        # "Update the current distance and then find the image closest to the desired distance and then display..."
                        n157 = call "RVHR - New Distance.vi"("Command"=enum16{"Next", "Previous"}."Next", "Local Data in"=w497, "UI Refs"=w491, "error in (no error)"=w499, "Supervisory Config Cluster In"=w494) -> ("error out"=w498:errorcluster, "Local Data out"=w496:T30)  [unwired: 4 in, 1 out]
                        n158 = call "RVHR - Get Current Images.vi"("Local Data in"=w496, "UI Refs"=w491, "error in (no error)"=w498) -> ("error out"=w492:errorcluster, "Local Data out"=w490:T30)  [unwired: 7 in]
                        n159 = call "Display Features.vi"("Local Data in"=w490, "UI References"=w491, "error in (no error)"=w492, "Action"=enum16{"All", "Preview", "Image"}."All") -> ("error out"=w488:errorcluster, "Local Data out"=w489:T30)  [unwired: 6 in]
                      }
                      frame "Previous Page" {
                        # "Update the current distance and then find the image closest to the desired distance and then display..."
                        n160 = call "RVHR - New Distance.vi"("Command"=enum16{"Next", "Previous"}."Previous", "Local Data in"=w509, "UI Refs"=w506, "error in (no error)"=w513, "Supervisory Config Cluster In"=w508) -> ("error out"=w512:errorcluster, "Local Data out"=w511:T30)  [unwired: 4 in, 1 out]
                        n161 = call "RVHR - Get Current Images.vi"("Local Data in"=w511, "UI Refs"=w506, "error in (no error)"=w512) -> ("error out"=w507:errorcluster, "Local Data out"=w505:T30)  [unwired: 7 in]
                        n162 = call "Display Features.vi"("Local Data in"=w505, "UI References"=w506, "error in (no error)"=w507, "Action"=enum16{"All", "Preview", "Image"}."All") -> ("error out"=w504:errorcluster, "Local Data out"=w503:T30)  [unwired: 6 in]
                      }
                      frame "Update Settings" {
                        # "Replot data relative to Users new settings..."
                        n163 = call "RVHR - Settings.vi"("error in (no error)"=w526) -> ("Error"=w520:errorcluster, "Cancelled?"=w521:bool, "Supervisory Config Cluster In"=w519:T9)  [unwired: 8 in]
                        n164 = case shown="False" w521 {
                          tunnel: w520 -> [w533 w537]
                          tunnel: w519 -> [w535 _]
                          tunnel: w524 -> [w534 w538]
                          tunnel: w523 -> [w527 _]
                          tunnel: [w529 w538] -> w525
                          tunnel: [w531 w537] -> w522
                          tunnel: [w535 w536] -> w518
                          tunnel: w517 -> [_ w536]
                          tunnel: w516 -> [_ _]
                          frame False {
                            # "Update settings and then refresh UI..."
                            n165 = call "RVHR - Get Current Images.vi"("Local Data in"=w534, "UI Refs"=w527, "error in (no error)"=w533) -> ("error out"=w532:errorcluster, "Local Data out"=w530:T30)  [unwired: 7 in]
                            n166 = call "Display Features.vi"("Local Data in"=w530, "UI References"=w527, "error in (no error)"=w532, "Action"=enum16{"All", "Preview", "Image"}."Image") -> ("error out"=w531:errorcluster, "Local Data out"=w529:T30)  [unwired: 6 in]
                          }
                          frame True {
                            # "Cancelled. So do nothing..."
                          }
                        }
                      }
                      frame "Image Processing" {
                        # "Display Image Processing Modal and then replot data..."
                        n167 = disable-structure shown="Disabled" {
                          disable-tunnel: [w566 w568] -> w547
                          disable-tunnel: w546 -> [w565 _]
                          disable-tunnel: [w564 w567] -> w545
                          disable-tunnel: w543 -> [w563 _]
                          disable-tunnel: w542 -> [w554 w568]
                          disable-tunnel: w541 -> [w550 w567]
                          frame Disabled {
                            n168 = Unbundle By Name(w565) -> ("Run Distance"=w561:refnum<vi>)
                            n169 = property class="Slide (strict)"(reference=w561, error in=w550) -> (error out=w549:errorcluster, "Value"=w560:cluster{dbl, dbl, dbl})  [unwired: 1 out]
                            n170 = Unbundle(w560) -> (w548:dbl)  [unwired: 2 out]
                            n171 = call "Vision - Get Current Image Filename.vi"("Current Position"=w548, "error in (no error)"=w549, "Local Data"=w554) -> ("error out"=w552:errorcluster, "Image Folder out"=w553:path)  [unwired: 7 in]
                            n172 = call "Image Processing.vi"("error in (no error)"=w552, "path to PNG file"=w553) -> ("error out"=w562:errorcluster)  [unwired: 9 in]
                            n173 = call "Vision - Calculate total Pages.vi"("Local Data in"=w554, "error in (no error)"=w562) -> ("error out"=w559:errorcluster, "Local Data out"=w557:T35)  [unwired: 8 in]
                            n174 = call "Vision - Sections UI.vi"("Local Data in"=w557, "error in (no error)"=w559) -> ("error out"=w558:errorcluster, "Local Data out"=w556:T35)  [unwired: 8 in]
                            n175 = call "Vision - Update Page.vi"("Local Data in"=w556, "error in (no error)"=w558, "Language Config Cluster"=w563) -> ("error out"=w551:errorcluster, "Local Data out"=w555:T35)  [unwired: 7 in]
                            n176 = call "Vision - Get Current Images.vi"("Local Data in"=w555, "error in (no error)"=w551, "Current Distance"=w548) -> ("error out"=w564:errorcluster, "Local Data out"=w566:T35)  [unwired: 7 in]
                          }
                          frame Enabled {
                          }
                        }
                      }
                      frame "Analysis" {
                        # "init python script running in background on startup\nWrite to trigger.csv file in appdata to start analysis"
                        # "1. select images to analyse - NT /\n2. create images.csv file - GM /\n3. call exe for analysis - GM /\n4. display progress - NT /\n5. if cancelled taskkill? - NT\n6a. results into results.csv - GM /\n6b. results into db NT /\n7. display results - NT \n8. save results csv with images? - DK"
                        # "ML Analysis - Not called (see machine learning loop below)"
                        n177 = disable-structure shown="Disabled" {
                          disable-tunnel: w576 -> [w596 w625 w646]
                          disable-tunnel: [w594 w608 w646] -> w575
                          disable-tunnel: w574 -> [w585 w624 _]
                          disable-tunnel: w573 -> [w584 w623 _]
                          disable-tunnel: w572 -> [_ w619 w644]
                          disable-tunnel: w571 -> [_ w618 w645]
                          disable-tunnel: [_ w617 w644] -> w570
                          disable-tunnel: [_ w616 w645] -> w569
                          frame Disabled {
                            w581 = ".db" ("replace string (\"\")")
                            n178 = Unbundle By Name(w585) -> ("Main Test Cluster.Path"=w595:path)
                            n179 = Strip Path(path=w595) -> (stripped path=w583:path, name=w593:string)
                            n180 = disable-structure shown="Enabled" {
                              disable-tunnel: w596 -> [w600 w605]
                              disable-tunnel: w583 -> [w599 _]
                              disable-tunnel: [w598 w604] -> w590
                              disable-tunnel: [w597 w603] -> w587
                              disable-tunnel: w585 -> [_ w602]
                              disable-tunnel: w584 -> [_ w601]
                              frame Disabled {
                                n181 = call "Multi Folder Select.vi"("error in"=w600, "Root Folder Path"=w599) -> ("error out"=w598:errorcluster, "Tags"=w597:string[])  [unwired: 8 in]
                              }
                              frame Enabled {
                                n182 = call "Current File Paths.vi"("Local Data in"=w602, "UI Refs"=w601, "error in (no error)"=w605) -> ("error out"=w604:errorcluster, "Tags"=w603:string[])  [unwired: 6 in, 1 out]
                              }
                            }
                            n183 = Strip Path(path=w583) -> (stripped path=w579:path, name=w582:string)
                            n184 = Concatenate Strings(w582, w581) -> (w580:string)
                            n185 = Search and Replace String(input string=w593, search string=".rvhr", replace string=w581, error in=w590) -> (result string=w591:string, error out=w589:errorcluster)  [unwired: 4 in, 2 out]
                            n186 = Build Path(base path=w579, name or relative path=w580) -> (appended path=w578:path)
                            n187 = Build Path(base path=w583, name or relative path=w591) -> ()  [unwired: 1 out]
                            n188 = call "run_model.vi"("error in (no error)"=w589, "Image Paths"=w587) -> ("error out"=w588:errorcluster, "Results path"=w586:path)  [unwired: 8 in]
                            n189 = call "csv-db.vi"("db path"=w578, "error in (no errror)"=w588, "results path"=w586) -> ("error out"=w594:errorcluster)  [unwired: 8 in]
                          }
                          frame Disabled {
                            n190 = Unbundle By Name(w624) -> ("Main Test Cluster.Path"=w607:path)
                            n191 = Strip Path(path=w607) -> (stripped path=w606:path)  [unwired: 1 out]
                            n192 = Strip Path(path=w606) -> (name=w622:string)  [unwired: 1 out]
                            n193 = disable-structure shown="Enabled" {
                              disable-tunnel: w625 -> [w638 w643]
                              disable-tunnel: [w637 w642] -> w608
                              disable-tunnel: [w636 w641] -> w620
                              disable-tunnel: w624 -> [_ w640]
                              disable-tunnel: w623 -> [_ w639]
                              frame Disabled {
                                n194 = call "Multi Folder Select.vi"("error in"=w638) -> ("error out"=w637:errorcluster, "Tags"=w636:string[])  [unwired: 9 in]
                              }
                              frame Enabled {
                                n195 = call "Current File Paths.vi"("Local Data in"=w640, "UI Refs"=w639, "error in (no error)"=w643) -> ("error out"=w642:errorcluster, "Tags"=w641:string[])  [unwired: 6 in, 1 out]
                              }
                            }
                            n196 = call <vilib>:"Application Directory.vi"() -> ("Application Directory"=w611:path)
                            n197 = Concatenate Strings(w622, ".db" ("replace string (\"\")")) -> (w621:string)
                            n198 = Build Path(base path=w611, name or relative path=path "Analysis/best.pt") -> (appended path=w610:path)
                            n199 = Build Path(base path=w606, name or relative path=w621) -> (appended path=w614:path)
                            n200 = Path To String(path=w614) -> (string=w613:string)
                            n201 = Path To String(path=w610) -> (string=w609:string)
                            n202 = for {
                              tunnel: w620 -> [w628] mode=indexing
                              shift-right: [w633] -> w616
                              shift-left: w618 -> [w631]
                              shift-right: [w634] -> w617
                              shift-left: w619 -> [w635]
                              tunnel: w613 -> [w627]
                              tunnel: w609 -> [w626]
                              # "for each image"
                              n203 = Format Into String(format string="ANALYSE,\"%s\",\"%s\",\"%s\"" ("replace string (\"\")"), error in=w631, w628, w626, w627) -> (resulting string=w629:string, error out=w630:errorcluster)  [unwired: 1 in]
                              n204 = call "send_command.vi"("error in (no error)"=w630, "command"=w629, "connection ID"=w635) -> ("error out"=w633:errorcluster, "connection ID out"=w634:refnum<k5>)  [unwired: 6 in, 1 out]
                            }
                          }
                          frame Enabled {
                          }
                        }
                      }
                      frame "Print Feature Report" {
                        # "Leave in!! Without this above printed report has a weird grey bar across\nthe bottom"
                        # "Print either the current page or a full report using the page distance to jog through the run..."
                        n205 = disable-structure shown="Enabled" {
                          disable-tunnel: w655 -> [w664 w669]
                          disable-tunnel: w656 -> [w663 w668]
                          disable-tunnel: Print_Command."Current Page" ("Command") -> [w662 _]
                          disable-tunnel: w653 -> [w661 _]
                          disable-tunnel: [w660 w667] -> w652
                          disable-tunnel: [w659 _] -> w651
                          disable-tunnel: w650 -> [w658 w670]
                          disable-tunnel: w649 -> [w657 _]
                          frame Disabled {
                            n206 = Current VI's Path() -> (path=w659:path)
                            n207 = call "RVHR - Print Report_ExaPromPDF.vi"("Main VI Path"=w659, "Settings"=w657, "Local Data"=w664, "UI Refs"=w658, "error in (no error)"=w663, "Language Config Cluster"=w661, "Command"=w662) -> ("error out"=w660:errorcluster)  [unwired: 4 in]
                            n208 = disable-structure shown="Disabled" {
                              disable-tunnel: w659 -> [w666 _]
                              frame Disabled {
                                n209 = Path To String(path=w666) -> (string=w665:string)
                                n210 = One Button Dialog(message=w665) -> ()  [unwired: 1 in, 1 out]
                              }
                              frame Enabled {
                              }
                            }
                          }
                          frame Enabled {
                            n211 = call "Print Features Report.vi"("Local Data in"=w669, "UI References"=w670, "error in (no error)"=w668) -> ("error out"=w667:errorcluster)  [unwired: 8 in]
                          }
                        }
                        n212 = disable-structure shown="Disabled" {
                          disable-tunnel: w651 -> [w677 _]
                          frame Disabled {
                            n213 = Open VI Reference(vi path=w677) -> (vi reference=w676:refnum<vi>)  [unwired: 5 in, 1 out]
                            n214 = invoke class="VI" method="FP.Get Image"(reference=w676, "visible area only"=TRUE ("Visible Area Only"), "image depth"=24 ("Image Depth")) -> ("image data"=w673:T40)  [unwired: 3 in, 5 out]
                            n215 = call <vilib>:"Draw Flattened Pixmap.vi"("image data"=w673, "picture"=picture data[5B]) -> ("new picture"=→"new picture":picture)  [unwired: 7 in]
                          }
                          frame Enabled {
                          }
                        }
                      }
                      frame "Exit" {
                        # "Save cut-out info for the current main run to its .cut file..."
                        n216 = disable-structure shown="Enabled" {
                          disable-tunnel: _ -> [w691 _]
                          disable-tunnel: w680 -> [w690 _]
                          disable-tunnel: [w689 _] -> w684
                          disable-tunnel: w683 -> [w688 w692]
                          disable-tunnel: [w687 w692] -> w682
                          frame Disabled {
                            n217 = call "Cut-Out File Manager.vi"("Local Data in"=w688, ".ini Controller"=enum16{"Read", "Write"}."Write", "error in (no error)"=w690, "Run Path"=w691) -> ("error out"=w689:errorcluster, "Local Data out"=w687:T41)  [unwired: 6 in]
                          }
                          frame Enabled {
                          }
                        }
                      }
                    }
                    n218 = call "Local Data FGV.vi"("Action"=enum16{"Set", "Get"}."Set", "Local Data"=w230) -> ("Local Data 2"=w229:T30)  [unwired: 9 in]
                    n219 = call "Handle Error.vi"("Clear Error?"=w240, "base path"=w239, "Command"=Error_Command."Handle", "error in (no error)"=w245, "Section of Code"=w242, "Test Name"="RV-HR_Reporting") -> ("error out"=w244:errorcluster)  [unwired: 3 in, 2 out]
                  }
                  n220 = while {
                    tunnel: w128 -> [w708]
                    tunnel: w141 -> [w706]
                    tunnel: w139 -> [w705]
                    tunnel: w138 -> [w698]
                    tunnel: w142 -> [w697]
                    shift-right: [w699] -> _
                    shift-left: w140 -> [w707]
                    shift-right: [w696] -> _
                    shift-left: _ -> [w695]
                    tunnel: w129 -> [w694]
                    tunnel: w127 -> [w693]
                    stop <- w709 stop-if-true
                    w702 = TRUE  # Clear Error?
                    # "Actions Handler"
                    n221 = event shown="[14] Menu Selection (User)" {
                      selector: _ -> [_ _ _ _ _ _ _ _ _ _ _ _ _ _ _ _ _ _ _ _ _ _]
                      dyn-events: _ -> [_ _ _ _ _ _ _ _ _ _ _ _ _ _ _ _ _ _ _ _ _ _]
                      timeout: _ -> [_ _ _ _ _ _ _ _ _ _ _ _ _ _ _ _ _ _ _ _ _ _]
                      tunnel: [_ _ _ _ _ _ _ _ _ _ _ _ _ _ w934 _ _ _ _ _ _ w1081] -> w709
                      tunnel: w708 -> [_ w715 w721 _ _ w754 _ _ w852 _ _ _ _ _ w939 w1025 w1033 w1038 w1051 w1063 w1072 w1080]
                      tunnel: w707 -> [w710 w716 w722 w725 w741 w755 w823 w841 w849 w890 w911 w917 w923 w927 w938 w1024 w1032 w1044 w1055 w1066 w1071 w1079]
                      tunnel: [w710 w711 w717 w724 w740 w753 w826 w840 w851 w889 w910 w916 w922 w926 w937 w1026 w1028 w1039 w1050 w1062 w1068 w1078] -> w701
                      tunnel: w706 -> [_ _ _ _ _ _ _ _ _ _ _ _ _ _ w935 _ _ _ _ _ _ _]
                      tunnel: w705 -> [_ _ _ w726 _ _ w820 _ _ _ w913 w919 w925 _ w932 _ _ _ _ w1060 _ w1076]
                      tunnel: w697 -> [_ _ _ _ w739 _ _ _ _ _ _ _ _ _ w931 _ _ _ _ _ _ _]
                      tunnel: [_ _ _ _ _ _ w818 _ _ _ _ _ _ _ _ _ _ _ _ _ _ _] -> w696
                      tunnel: w695 -> [_ _ _ _ _ _ w817 _ _ _ _ _ _ _ _ _ _ _ _ _ _ _]
                      tunnel: w694 -> [_ _ _ _ _ _ _ _ _ _ _ _ _ w928 w933 _ _ _ _ _ _ w1077]
                      tunnel: w693 -> [_ _ _ _ _ _ _ _ _ _ _ _ _ _ w930 _ _ _ _ _ _ _]
                      event Timeout {
                        n222 = event-data() -> ()  [unwired: 1 in, 1 out]
                      }
                      event "Next?": Value Change {
                        # "Transition to next page..."
                        n223 = event-data() -> ("CtlRef"=w712:refnum<vi>)  [unwired: 1 in]
                        n224 = Enqueue Element(queue=w715, element=cluster{"Command":string, "Data":variant} {"Command"="Next Page", "Data"=variant} ("output cluster"), error in (no error)=w716) -> (error out=w713:errorcluster)  [unwired: 1 in, 2 out]
                        n225 = call "Pop Button back up.vi"("error in (no error)"=w713, "Boolean in"=w712) -> ("error out"=w711:errorcluster)  [unwired: 9 in]
                      }
                      event "Previous?": Value Change {
                        # "Transition to previous page..."
                        n226 = event-data() -> ("CtlRef"=w718:refnum<vi>)  [unwired: 1 in]
                        n227 = Enqueue Element(queue=w721, element=cluster{"Command":string, "Data":variant} {"Command"="Previous Page", "Data"=variant} ("output cluster"), error in (no error)=w722) -> (error out=w719:errorcluster)  [unwired: 1 in, 2 out]
                        n228 = call "Pop Button back up.vi"("error in (no error)"=w719, "Boolean in"=w718) -> ("error out"=w717:errorcluster)  [unwired: 9 in]
                      }
                      event Key Down {
                        # "Catch Left and Right key down events and tie to the UI Next and Previous buttons..."
                        n229 = event-data() -> ("VKey"=w723:T42)  [unwired: 1 in]
                        n230 = case shown="\"Left\"" w723 {
                          tunnel: w725 -> [w727 w731 w736]
                          tunnel: w726 -> [_ w732 w737]
                          tunnel: [w727 w728 w733] -> w724
                          frame "ASCII", Default {
                          }
                          frame "Left" {
                            n231 = Unbundle By Name(w732) -> ("Previous?"=w730:refnum<vi>)
                            n232 = property class="Bool (strict)"(reference=w730, error in=w731, "Val(Sgnl)"=TRUE ("Value (Signaling)")) -> (error out=w728:errorcluster)  [unwired: 1 out]
                          }
                          frame "Right" {
                            n233 = Unbundle By Name(w737) -> ("Next?"=w735:refnum<vi>)
                            n234 = property class="Bool (strict)"(reference=w735, error in=w736, "Val(Sgnl)"=TRUE ("Value (Signaling)")) -> (error out=w733:errorcluster)  [unwired: 1 out]
                          }
                        }
                      }
                      event "Image": Shortcut Menu Activation? {
                        # "USE IF NEED TO ADD A RUNTIME MENU FOR ADDING FEATURES ETC."
                        # "Configure the short cut menu before presented to the user..."
                        n235 = event-data() -> ("MenuRef"=w738:refnum<k9>)  [unwired: 1 in]
                        n236 = disable-structure shown="Enabled" {
                          disable-tunnel: w741 -> [w748 w750]
                          disable-tunnel: [w747 w750] -> w740
                          disable-tunnel: w739 -> [w746 _]
                          disable-tunnel: w738 -> [w743 _]
                          frame Enabled {
                            n237 = Unbundle By Name(w746) -> ("Remove Feature"=w745:string)
                            n238 = Build Array(w745, "Edit Feature Type" ("element")) -> (w744:string[])
                            n239 = Insert Menu Items(6:w748, 7:string[] ["USER_Remove", "USER_Edit"] ("item names"), 8:w744, 9:w743) -> (0:w747:errorcluster)  [unwired: 2 in, 2 out]
                          }
                          frame Disabled {
                          }
                        }
                        n240 = event-data() -> ()  [unwired: 2 in, 1 out]
                      }
                      event "Image": Shortcut Menu Selection (User) {
                        # "Register the SC selection and act upon it..."
                        n241 = event-data() -> ("CtlRef"=w756:refnum<vi>, "ItemTag"=w751:string, "Coords"=w752:T16)  [unwired: 1 in, 2 out]
                        n242 = disable-structure shown="Enabled" {
                          disable-tunnel: w756 -> [w762 w797]
                          disable-tunnel: w755 -> [w761 w796]
                          disable-tunnel: w754 -> [w760 w795]
                          disable-tunnel: [w759 w794] -> w753
                          disable-tunnel: w752 -> [w757 w792]
                          disable-tunnel: w751 -> [w758 w793]
                          frame Enabled {
                            n243 = case shown="\"USER_Edit\"" w758 {
                              tunnel: w762 -> [_ w773 w787]
                              tunnel: w761 -> [w763 w769 w783]
                              tunnel: w760 -> [_ w777 w791]
                              tunnel: [w763 w766 w780] -> w759
                              tunnel: w757 -> [_ _ _]
                              frame "0", Default {
                              }
                              frame "USER_Remove" {
                                # "User selection. Send to consumer."
                                n244 = property class="Pict"(reference=w773, error in=w769) -> ("Mouse"=w772:T43)  [unwired: 2 out]
                                n245 = property class="Pict"(reference=w773, error in=w769) -> (error out=w768:errorcluster, "Label.Text"=w771:string)  [unwired: 1 out]
                                n246 = Unbundle By Name(w772) -> ("Mouse Position"=w770:cluster{"X":i32, "Y":i32})
                                n247 = Bundle("Label.Text"=w771, "Mouse Position"=w770) -> (w774:T44)  [unwired: 1 in]
                                n248 = Bundle By Name(cluster=cluster{"Command":string, "Data":variant} {"Command"="Remove Feature", "Data"=variant} ("output cluster"), "Data"=w774) -> (w775:cluster{"Command":string, "Data":variant})
                                n249 = Enqueue Element(queue=w777, element=w775, error in (no error)=w768) -> (queue out=w765:refnum<queue>, error out=w767:errorcluster)  [unwired: 1 in, 1 out]
                                n250 = Enqueue Element(queue=w765, element=cluster{"Command":string, "Data":variant} {"Command"="Refresh Plot", "Data"=variant} ("output cluster"), error in (no error)=w767) -> (error out=w766:errorcluster)  [unwired: 1 in, 2 out]
                              }
                              frame "USER_Edit" {
                                # "User selection. Send to consumer."
                                n251 = property class="Pict"(reference=w787, error in=w783) -> ("Mouse"=w786:T43)  [unwired: 2 out]
                                n252 = property class="Pict"(reference=w787, error in=w783) -> (error out=w782:errorcluster, "Label.Text"=w785:string)  [unwired: 1 out]
                                n253 = Unbundle By Name(w786) -> ("Mouse Position"=w784:cluster{"X":i32, "Y":i32})
                                n254 = Bundle("Label.Text"=w785, "Mouse Position"=w784) -> (w788:T44)  [unwired: 1 in]
                                n255 = Bundle By Name(cluster=cluster{"Command":string, "Data":variant} {"Command"="Edit Feature", "Data"=variant} ("output cluster"), "Data"=w788) -> (w789:cluster{"Command":string, "Data":variant})
                                n256 = Enqueue Element(queue=w791, element=w789, error in (no error)=w782) -> (queue out=w779:refnum<queue>, error out=w781:errorcluster)  [unwired: 1 in, 1 out]
                                n257 = Enqueue Element(queue=w779, element=cluster{"Command":string, "Data":variant} {"Command"="Refresh Plot", "Data"=variant} ("output cluster"), error in (no error)=w781) -> (error out=w780:errorcluster)  [unwired: 1 in, 2 out]
                              }
                            }
                          }
                          frame Disabled {
                            n258 = case shown="\"USER_Remove\"" w793 {
                              tunnel: w797 -> [_ w799]
                              tunnel: w796 -> [w798 w812]
                              tunnel: w795 -> [_ w811]
                              tunnel: [w798 w806] -> w794
                              tunnel: w792 -> [_ w800]
                              frame "0", Default {
                              }
                              frame "USER_Remove" {
                                # "User selection. Send to consumer."
                                n259 = invoke class="Pict" method="Map Coords To XY"(reference=w799, error in=w812, "Coords"=w800) -> (error out=w810:errorcluster, "XY"=w807:cluster{"X":dbl, "Y":dbl})  [unwired: 4 in, 5 out]
                                n260 = property class="Pict"(reference=w799) -> ("Label.Text"=w802:string)  [unwired: 1 in, 2 out]
                                n261 = Unbundle By Name(w807) -> ("X"=w805:dbl)
                                n262 = String Subset(string=w802, length (rest)=5 ("length (rest)")) -> (substring=w801:string)  [unwired: 1 in]
                                n263 = Bundle("X"=w805, "Label.Text"=w801) -> (w804:cluster{"X":dbl, "Label.Text":string})  [unwired: 1 in]
                                n264 = Bundle By Name(cluster=cluster{"Command":string, "Data":variant} {"Command"="Remove Cut-Out", "Data"=variant} ("output cluster"), "Data"=w804) -> (w808:cluster{"Command":string, "Data":variant})
                                n265 = Enqueue Element(queue=w811, element=w808, error in (no error)=w810) -> (error out=w806:errorcluster)  [unwired: 1 in, 2 out]
                              }
                            }
                          }
                        }
                      }
                      event "Image": Mouse Move {
                        # "Zoom window pop up"
                        n266 = event-data() -> ("CtlRef"=w813:refnum<vi>)  [unwired: 1 in, 4 out]
                        n267 = Tick Count (ms)() -> (millisecond timer value=w819:u32)
                        n268 = Subtract(x=w819, y=w817) -> (x-y=w825:u32)
                        n269 = call "Draw Feature Box.vi"("Action"=enum16{"Mouse Move", "Mouse Down", "Mouse Up"}."Mouse Move", "error in (no error)"=w823, "UI References"=w820, "CtlRef"=w813) -> ("error out"=w822:errorcluster)  [unwired: 5 in, 2 out]
                        n270 = Greater?(x=w825, y=u32 10) -> (0:w815:bool)
                        n271 = And(x="Zoom Window", y=w815) -> (x .and. y?=w814:T6)
                        n272 = case shown="True" w814 {
                          tunnel: w813 -> [_ w834]
                          tunnel: w822 -> [w828 w832]
                          tunnel: [w828 w837] -> w826
                          tunnel: w819 -> [_ w829]
                          tunnel: [w827 w829] -> w818
                          tunnel: w817 -> [w827 _]
                          frame False {
                          }
                          frame True {
                            n273 = property class="Pict"(reference=w834, error in=w832) -> (reference out=w830:refnum<vi>, error out=w831:errorcluster, "Mouse"=w833:T43)
                            n274 = Unbundle By Name(w833) -> ("Mouse Position"=w835:cluster{"X":i32, "Y":i32})
                            n275 = call "Zoom Window.vi"("window size"=100, "error in (no error)"=w831, "Mouse Position"=w835, "CtlRef"=w830) -> ("error out"=w837:errorcluster)  [unwired: 7 in]
                          }
                        }
                      }
                      event "Image": Mouse Down {
                        # "now checking if scrollbars are beng used."
                        n276 = event-data() -> ("Button"=w839:u16, "CtlRef"=w838:refnum<vi>)  [unwired: 1 in]
                        n277 = case shown="1" w839 {
                          tunnel: w838 -> [_ w846 _]
                          tunnel: w841 -> [w842 w845 w847]
                          tunnel: [w842 w844 w847] -> w840
                          frame 0, Default {
                          }
                          frame 1 {
                            # "Left mouse click"
                            n278 = call "Draw Feature Box.vi"("Action"=enum16{"Mouse Move", "Mouse Down", "Mouse Up"}."Mouse Down", "error in (no error)"=w845, "CtlRef"=w846) -> ("error out"=w844:errorcluster)  [unwired: 6 in, 2 out]
                          }
                          frame 2 {
                            # "Right mouse click"
                          }
                        }
                      }
                      event "Image": Mouse Up {
                        # "using the scrollbars is triggering mouse down.\nmouse move, mouse up events. In the mouse\nup event, if 'can add?' is False, a 'Refresh Plot'\nevent is queued causing the image to zoom\nout."
                        n279 = event-data() -> ("CtlRef"=w850:refnum<vi>, "Button"=w848:u16)  [unwired: 1 in, 6 out]
                        n280 = case shown="1" w848 {
                          tunnel: w852 -> [_ w863 _]
                          tunnel: [w853 w861 w887] -> w851
                          tunnel: w850 -> [_ w857 _]
                          tunnel: w849 -> [w853 w856 w887]
                          frame 0, Default {
                          }
                          frame 1 {
                            # "Left mouse click"
                            n281 = property class="Pict"(reference=w857, error in=w856) -> (reference out=w858:refnum<vi>, error out=w855:errorcluster, "Label.Text"=w860:string)
                            n282 = call "Draw Feature Box.vi"("Action"=enum16{"Mouse Move", "Mouse Down", "Mouse Up"}."Mouse Up", "error in (no error)"=w855, "CtlRef"=w858) -> ("error out"=w862:errorcluster, "Can Add?"=w854:bool, "Mouse Position (Start)"=w859:cluster{"X":i32, "Y":i32})  [unwired: 6 in]
                            n283 = case shown="True" w854 {
                              tunnel: w863 -> [w872 w877]
                              tunnel: w862 -> [w871 w876]
                              tunnel: [w870 w875] -> w861
                              tunnel: w860 -> [w867 w874]
                              tunnel: w859 -> [w866 w873]
                              frame True {
                                # "Valid, so add FTR"
                                n284 = Bundle("Label.Text"=w867, "Mouse Position (Start)"=w866) -> (w865:T14)  [unwired: 1 in]
                                n285 = Bundle By Name(cluster=cluster{"Command":string, "Data":variant} {"Command"="Add Feature", "Data"=variant} ("output cluster"), "Data"=w865) -> (w869:cluster{"Command":string, "Data":variant})
                                n286 = Enqueue Element(queue=w872, element=w869, error in (no error)=w871) -> (error out=w870:errorcluster)  [unwired: 1 in, 2 out]
                              }
                              frame False {
                                # "Remove overlay"
                                n287 = disable-structure shown="Disabled" {
                                disable-tunnel: w877 -> [w885 _]
                                disable-tunnel: w876 -> [w884 w886]
                                disable-tunnel: [w883 w886] -> w875
                                disable-tunnel: w874 -> [w880 _]
                                disable-tunnel: w873 -> [w879 _]
                                frame Disabled {
                                n288 = Bundle("Label.Text"=w880, "Mouse Position (Start)"=w879) -> (w878:T14)  [unwired: 1 in]
                                n289 = Bundle By Name(cluster=cluster{"Command":string, "Data":variant} {"Command"="Refresh Plot", "Data"=variant} ("output cluster"), "Data"=w878) -> (w882:cluster{"Command":string, "Data":variant})
                                n290 = Enqueue Element(queue=w885, element=w882, error in (no error)=w884) -> (error out=w883:errorcluster)  [unwired: 1 in, 2 out]
                                }
                                frame Enabled {
                                # "remove bad feature\nif drawn?"
                                }
                                }
                              }
                            }
                          }
                          frame 2 {
                            # "Right mouse click"
                          }
                        }
                      }
                      event Value Change {
                        n291 = event-data() -> ("NewVal"=w888:T6)  [unwired: 1 in, 5 out]
                        n292 = disable-structure shown="Enabled" {
                          disable-tunnel: [w896 "Zoom Window.vi"] -> w891
                          frame Disabled {
                            n293 = call <vilib>:"Application Directory.vi"() -> ("Application Directory"=w898:path)
                            n294 = Build Path(base path=w898, name or relative path=path "SubVIs/Zoom Window.vi") -> (appended path=w896:path)
                          }
                          frame Enabled {
                          }
                        }
                        n295 = Open VI Reference(vi path=w891, error in (no error)=w890) -> (vi reference=w895:refnum<vi>, error out=w893:errorcluster)  [unwired: 4 in]
                        n296 = case shown="False" w888 {
                          tunnel: w895 -> [w903 w907]
                          tunnel: [w902 w906] -> w894
                          tunnel: w893 -> [w901 w905]
                          tunnel: [w900 w904] -> w892
                          frame True {
                            n297 = invoke class="VI" method="FP.Open"(reference=w903, error in=w901) -> (reference out=w902:refnum<vi>, error out=w900:errorcluster)  [unwired: 3 in, 3 out]
                          }
                          frame False {
                            n298 = invoke class="VI" method="FP.Close"(reference=w907, error in=w905) -> (reference out=w906:refnum<vi>, error out=w904:errorcluster)  [unwired: 1 in, 1 out]
                          }
                        }
                        n299 = Close Reference(reference=w894, error in (no error)=w892) -> (error out=w889:errorcluster)
                      }
                      event Value Change {
                        n300 = event-data() -> ()  [unwired: 1 in, 6 out]
                        n301 = Unbundle By Name(w913) -> ("Zoom Toolbar L"=w909:refnum<vi>, "Image"=w912:refnum<vi>)
                        n302 = call "Zoom Manager.vi"("Command"=enum16{"Zoom IN", "Zoom OUT", "Fit"}."Zoom OUT", "error in (no error)"=w911, "Image"=w912, "Zoom Cluster"=w909) -> ("error out"=w910:errorcluster)  [unwired: 7 in]
                      }
                      event Value Change {
                        n303 = event-data() -> ()  [unwired: 1 in, 6 out]
                        n304 = Unbundle By Name(w919) -> ("Zoom Toolbar L"=w915:refnum<vi>, "Image"=w918:refnum<vi>)
                        n305 = call "Zoom Manager.vi"("Command"=enum16{"Zoom IN", "Zoom OUT", "Fit"}."Zoom IN", "error in (no error)"=w917, "Image"=w918, "Zoom Cluster"=w915) -> ("error out"=w916:errorcluster)  [unwired: 7 in]
                      }
                      event Value Change {
                        n306 = event-data() -> ()  [unwired: 1 in, 6 out]
                        n307 = Unbundle By Name(w925) -> ("Zoom Toolbar L"=w921:refnum<vi>, "Image"=w924:refnum<vi>)
                        n308 = call "Zoom Manager.vi"("Command"=enum16{"Zoom IN", "Zoom OUT", "Fit"}."Fit", "error in (no error)"=w923, "Image"=w924, "Zoom Cluster"=w921) -> ("error out"=w922:errorcluster)  [unwired: 7 in]
                      }
                      event Value Change {
                        # "Start ML Analysis"
                        n309 = event-data() -> ()  [unwired: 1 in, 6 out]
                        n310 = Enqueue Element(queue=w928, element=cluster{"Command":string, "Data":variant} {"Command"="Analysis", "Data"=variant}, error in (no error)=w927) -> (error out=w926:errorcluster)  [unwired: 1 in, 2 out]
                      }
                      event Menu Selection (User) {
                        # "Handle RT Menu User Selections..."
                        n311 = event-data() -> ("ItemTag"=w936:string)  [unwired: 1 in]
                        n312 = case shown="\"Analyse All\"" w936 {
                          selector: w936 -> [w942 _ _ _ _ _ _ _ _]
                          tunnel: w939 -> [_ w950 w960 w961 _ _ w1011 w1018 w1022]
                          tunnel: w938 -> [w943 w947 w958 w963 w971 w992 w1012 w1016 w1020]
                          tunnel: [w943 w951 w959 w962 w976 w997 w1013 w1017 w1021] -> w937
                          tunnel: w935 -> [_ _ _ _ w968 w989 _ _ _]
                          tunnel: [_ _ _ _ _ _ TRUE _ _] -> w934
                          tunnel: w933 -> [_ _ _ _ w975 w996 w1010 _ _]
                          tunnel: w932 -> [_ _ _ _ w974 w995 w1009 _ _]
                          tunnel: w931 -> [_ _ _ _ w969 w990 _ _ _]
                          tunnel: w930 -> [_ _ _ _ w967 w988 _ _ _]
                          frame "False", Default {
                            n313 = Concatenate Strings("Run-Time Menu Selection:\n\n" ("string"), w942) -> (w941:string)
                            n314 = One Button Dialog(message=w941) -> ()  [unwired: 1 in, 1 out]
                          }
                          frame "Load New" {
                            # "Load a New Main Run..."
                            n315 = call "RVHR - File Selection.vi"("error in"=w947) -> ("error out"=w946:errorcluster, "cancelled?"=w944:bool, "RVHR path"=w945:path)  [unwired: 8 in]
                            n316 = Bundle By Name(cluster=cluster{"Command":string, "Data":variant} {"Command"="Process Main", "Data"=variant} ("output cluster"), "Data"=w945) -> (w948:cluster{"Command":string, "Data":variant})
                            n317 = case shown="False" w944 {
                              tunnel: w946 -> [w952 w956]
                              tunnel: w950 -> [w953 _]
                              tunnel: [w955 w956] -> w951
                              tunnel: w948 -> [w954 _]
                              frame False {
                                n318 = Enqueue Element(queue=w953, element=w954, error in (no error)=w952) -> (error out=w955:errorcluster)  [unwired: 1 in, 2 out]
                              }
                              frame True {
                              }
                            }
                          }
                          frame "Print Feature Report" {
                            # "Print a Feature report..."
                            n319 = Enqueue Element(queue=w960, element=cluster{"Command":string, "Data":variant} {"Command"="Print Feature Report", "Data"=variant} ("output cluster"), error in (no error)=w958) -> (error out=w959:errorcluster)  [unwired: 1 in, 2 out]
                          }
                          frame "Print All Pages" {
                            # "Print a full report..."
                            n320 = Bundle By Name(cluster=cluster{"Command":string, "Data":variant} {"Command"="Print", "Data"=variant} ("output cluster"), "Data"=Print_Command."Full Report" ("Command")) -> (w965:cluster{"Command":string, "Data":variant})
                            n321 = Enqueue Element(queue=w961, element=w965, error in (no error)=w963) -> (error out=w962:errorcluster)  [unwired: 1 in, 2 out]
                          }
                          frame "Analyse Current" {
                            # "Analyse Current images..."
                            n322 = Unbundle By Name(w974) -> ("ML Analysis"=w973:refnum<vi>)
                            n323 = property class="Bool (strict)"(reference=w973, error in=w971) -> (error out=w970:errorcluster, "DisabledEnum"=w972:T11)  [unwired: 1 out]
                            n324 = case shown="\"Disabled\"" w972 {
                              tunnel: w970 -> [w980 w985]
                              tunnel: [w979 w984] -> w976
                              tunnel: w975 -> [_ w983]
                              tunnel: w969 -> [w978 _]
                              tunnel: w968 -> [_ _]
                              tunnel: w967 -> [w977 _]
                              frame "Enabled", Default {
                                n325 = Unbundle By Name(w978) -> ("AI Not Ready"=w981:string)
                                n326 = call "Win Host - dialog_1bt.vi"("Language"=w977, "error in (no error)"=w980, "Message"=w981) -> ("error out"=w979:errorcluster)  [unwired: 7 in, 1 out]
                              }
                              frame "Disabled" {
                                n327 = Bundle By Name(cluster=cluster{"Command":string, "Data":variant} {"Command"="Analysis", "Data"=variant} ("output cluster"), "Data"=RVHR_-_Analysis_Mode."Current Images" ("Analysis Mode")) -> (w986:cluster{"Command":string, "Data":variant})
                                n328 = Enqueue Element(queue=w983, element=w986, error in (no error)=w985) -> (error out=w984:errorcluster)  [unwired: 1 in, 2 out]
                              }
                            }
                          }
                          frame "Analyse All" {
                            # "Analyse All Images..."
                            n329 = Unbundle By Name(w995) -> ("ML Analysis"=w994:refnum<vi>)
                            n330 = property class="Bool (strict)"(reference=w994, error in=w992) -> (error out=w991:errorcluster, "DisabledEnum"=w993:T11)  [unwired: 1 out]
                            n331 = case shown="\"Enabled\", Default" w993 {
                              tunnel: w991 -> [w1001 w1006]
                              tunnel: [w1000 w1005] -> w997
                              tunnel: w996 -> [_ w1004]
                              tunnel: w990 -> [w999 _]
                              tunnel: w989 -> [_ _]
                              tunnel: w988 -> [w998 _]
                              frame "Enabled", Default {
                                n332 = Unbundle By Name(w999) -> ("AI Not Ready"=w1002:string)
                                n333 = call "Win Host - dialog_1bt.vi"("Language"=w998, "error in (no error)"=w1001, "Message"=w1002) -> ("error out"=w1000:errorcluster)  [unwired: 7 in, 1 out]
                              }
                              frame "Disabled" {
                                n334 = Bundle By Name(cluster=cluster{"Command":string, "Data":variant} {"Command"="Analysis", "Data"=variant} ("output cluster"), "Data"=RVHR_-_Analysis_Mode."Full Run" ("Analysis Mode")) -> (w1007:cluster{"Command":string, "Data":variant})
                                n335 = Enqueue Element(queue=w1004, element=w1007, error in (no error)=w1006) -> (error out=w1005:errorcluster)  [unwired: 1 in, 2 out]
                              }
                            }
                          }
                          frame "Quit" {
                            # "Shut the software down..."
                            n336 = call "Exit Manager.vi"("error in (no error)"=w1012, "uI Refs"=w1009, "Analysis Queue"=w1010, "Consumer Queue"=w1011) -> ("error out"=w1013:errorcluster)  [unwired: 7 in]
                          }
                          frame "Settings" {
                            # "Display Settings Modal and Update if needed..."
                            n337 = Enqueue Element(queue=w1018, element=cluster{"Command":string, "Data":variant} {"Command"="Update Settings", "Data"=variant} ("output cluster"), error in (no error)=w1016) -> (error out=w1017:errorcluster)  [unwired: 1 in, 2 out]
                          }
                          frame "Image Processing" {
                            # "Display Image Processing Modal and then update..."
                            n338 = Enqueue Element(queue=w1022, element=cluster{"Command":string, "Data":variant} {"Command"="Image Processing", "Data"=variant} ("output cluster"), error in (no error)=w1020) -> (error out=w1021:errorcluster)  [unwired: 1 in, 2 out]
                          }
                        }
                      }
                      event "Run Start", "Run End": Value Change {
                        # "Handle User run distance changes and pass onto the consumer..."
                        n339 = event-data() -> ()  [unwired: 1 in, 1 out]
                        n340 = Enqueue Element(queue=w1025, element=cluster{"Command":string, "Data":variant} {"Command"="Update Run Distance", "Data"=variant} ("output cluster"), error in (no error)=w1024) -> (error out=w1026:errorcluster)  [unwired: 1 in, 2 out]
                      }
                      event "Run Distance": Value Change {
                        # "Update the image for the new distance..."
                        n341 = event-data() -> ("NewVal"=w1027:dbl)  [unwired: 1 in]
                        n342 = Bundle By Name(cluster=cluster{"Command":string, "Data":variant} {"Command"="Update Current Distance", "Data"=variant} ("output cluster"), "Data"=w1027) -> (w1030:cluster{"Command":string, "Data":variant})
                        n343 = Enqueue Element(queue=w1033, element=w1030, error in (no error)=w1032) -> (error out=w1029:errorcluster)  [unwired: 1 in, 2 out]
                        n344 = case shown="No Error" w1029 {
                          selector: w1029 -> [w1035 w1036]
                          tunnel: [w1035 w1036] -> w1028
                          frame No Error {
                            # "Limit # of Events"
                            n345 = Wait (ms)(milliseconds to wait=u32 50) -> ()  [unwired: 1 out]
                          }
                          frame Error {
                          }
                        }
                      }
                      event "Feature Type:": Value Change {
                        n346 = event-data() -> ("CtlRef"=w1043:refnum<vi>)  [unwired: 1 in]
                        n347 = property class="Ring (strict)"(reference=w1043, error in=w1044) -> (error out=w1040:errorcluster, "Strings []"=w1041:string[], "Value"=w1042:u16)  [unwired: 1 out]
                        n348 = Index Array(array=w1041, index=w1042) -> (element=w1037:string)
                        n349 = case shown="\"Add New...\"" w1037 {
                          tunnel: w1040 -> [w1045 w1049]
                          tunnel: [w1045 w1048] -> w1039
                          tunnel: w1038 -> [_ w1046]
                          frame "False", Default {
                          }
                          frame "Add New..." {
                            n350 = Enqueue Element(queue=w1046, element=cluster{"Command":string, "Data":variant} {"Command"="Add New feature Type", "Data"=variant} ("output cluster"), error in (no error)=w1049) -> (error out=w1048:errorcluster)  [unwired: 1 in, 2 out]
                          }
                        }
                      }
                      event "All?": Value Change {
                        n351 = event-data() -> ("NewVal"=w1054:bool)  [unwired: 1 in]
                        n352 = call "Win Host - Run List Manager.vi"("Command"=Run_Listbox_Command."Update All", "error in (no error)"=w1055, "All? IN"=w1054) -> ("error out"=w1052:errorcluster)  [unwired: 5 in, 3 out]
                        n353 = Enqueue Element(queue=w1051, element=cluster{"Command":string, "Data":variant} {"Command"="Refresh Plot", "Data"=variant} ("output cluster"), error in (no error)=w1052) -> (error out=w1050:errorcluster)  [unwired: 1 in, 2 out]
                      }
                      event "Run Selection Listbox": Mouse Down {
                        n354 = event-data() -> ("Coords"=w1061:T16)  [unwired: 1 in]
                        n355 = Unbundle By Name(w1060) -> ("All?"=w1058:refnum<vi>)
                        n356 = call "Win Host - Run List Manager.vi"("Point32"=w1061, "Command"=Run_Listbox_Command."Update", "error in (no error)"=w1066) -> ("error out"=w1064:errorcluster, "All? OUT"=w1057:bool)  [unwired: 5 in, 2 out]
                        n357 = property class="Bool (strict)"(reference=w1058, error in=w1064, "Value"=w1057) -> (error out=w1059:errorcluster)  [unwired: 1 out]
                        n358 = Enqueue Element(queue=w1063, element=cluster{"Command":string, "Data":variant} {"Command"="Refresh Plot", "Data"=variant} ("output cluster"), error in (no error)=w1059) -> (error out=w1062:errorcluster)  [unwired: 1 in, 2 out]
                      }
                      event Panel Resize {
                        # "Refresh the plot to ensure that the plot labels update..."
                        n359 = event-data() -> ()  [unwired: 1 in, 2 out]
                        n360 = Enqueue Element(queue=w1072, element=cluster{"Command":string, "Data":variant} {"Command"="Refresh Plot", "Data"=variant} ("output cluster"), error in (no error)=w1071) -> (error out=w1069:errorcluster)  [unwired: 1 in, 2 out]
                        n361 = case shown="No Error" w1069 {
                          selector: w1069 -> [w1074 w1075]
                          tunnel: [w1074 w1075] -> w1068
                          frame No Error {
                            n362 = Wait (ms)(milliseconds to wait=u32 1000) -> ()  [unwired: 1 out]
                          }
                          frame Error {
                          }
                        }
                      }
                      event Panel Close? {
                        w1081 = TRUE ("Discard?")
                        # "Exit Software..."
                        n363 = event-data() -> ()  [unwired: 1 in, 4 out]
                        n364 = call "Exit Manager.vi"("error in (no error)"=w1079, "uI Refs"=w1076, "Analysis Queue"=w1077, "Consumer Queue"=w1080) -> ("error out"=w1078:errorcluster)  [unwired: 7 in]
                        n365 = event-data("Discard?"=w1081) -> ()  [unwired: 1 in, 1 out]
                      }
                    }
                    n366 = call "Handle Error.vi"("Clear Error?"=w702, "base path"=w698, "Command"=Error_Command."Handle", "error in (no error)"=w701, "Section of Code"="Events", "Test Name"="RV-HR_Reporting") -> ("error out"=w699:errorcluster)  [unwired: 3 in, 2 out]
                  }
                  n367 = disable-structure shown="Disabled" {
                    frame Disabled {
                      # "Display"
                      n368 = call "Zoom Window.vi"() -> ()  [unwired: 11 in, 1 out]
                      n369 = call "Get Features DB.vi"() -> ()  [unwired: 7 in, 5 out]
                      n370 = call "Preview.vi"() -> ()  [unwired: 10 in, 2 out]
                      n371 = call "Display Feature Preview.vi"() -> ()  [unwired: 11 in, 1 out]
                      n372 = call "Preview Pop Up.vi"() -> ()  [unwired: 10 in, 2 out]
                      n373 = call "Display Image Features.vi"() -> ()  [unwired: 11 in, 1 out]
                      n374 = call "Display Features.vi"() -> ()  [unwired: 10 in, 2 out]
                    }
                    frame Enabled {
                    }
                  }
                }
                frame Error {
                  n375 = Unbundle By Name(w1085) -> ("Language"=w1084:T19)
                  n376 = Unbundle By Name(w1087) -> ("Run Load Error"=w1086:string)
                  n377 = Unbundle By Name(w1090) -> ("source"=w1089:string)
                  n378 = Concatenate Strings(w1086, w1089) -> (w1088:string)
                  n379 = call "Win Host - dialog.vi"("Language"=w1084, "Message"=w1088) -> ()  [unwired: 8 in, 2 out]
                }
              }
              n380 = Release Queue(queue=w108, error in (no error)=w107) -> (error out=w104:errorcluster)  [unwired: 1 in, 2 out]
              n381 = Release Queue(queue=w74, error in (no error)=w75) -> ()  [unwired: 1 in, 3 out]
            }
            frame True {
              # "Error 43 occurred at File Dialog->Main.vi\n\nPossible reason(s):\n\nLabVIEW:  Operation cancelled by user."
              # "Cancelled. so do nothing."
              n382 = call <vilib>:"Clear Errors.vi"("error in (no error)"=w1095, "specific error code to clear (0: all)"=43) -> ("error out"=w1094:errorcluster)  [unwired: 4 in, 1 out]
            }
          }
        }
        frame True {
          # "Calncelled... so do nothing and return to main VI."
        }
      }
    }
    frame Error {
      n383 = Unbundle By Name(w1098) -> ("source"=w1101:string)
      n384 = Concatenate Strings("Report Loading Error:\n" ("string"), w1101) -> (w1099:string)
      n385 = call "Win Host - dialog.vi"("Language"=Language."English", "Message"=w1099) -> ()  [unwired: 8 in, 2 out]
    }
  }
  n386 = call "Taskkill.vi"("error in (no error)"=w5) -> ("error out"=w4:errorcluster)  [unwired: 9 in, 1 out]
  n387 = call "Empty TEMP Folder.vi"("error in (no error)"=w4) -> ("error out"=w3:errorcluster)  [unwired: 9 in, 1 out]
  n388 = call <vilib>:"Clear Errors.vi"("error in (no error)"=w3) -> ("error out"=w1:errorcluster)  [unwired: 5 in, 1 out]
  n389 = control-ref of="This Application"() -> (w10:refnum<vi>)
  n390 = property class="App"(reference=w10, error in=w1) -> (error out=w11:errorcluster, "App.Kind"=w2:T45)  [unwired: 1 out]
  n391 = case shown="\"Run Time System\"" w2 {
    tunnel: w11 -> [w1102 w1103 w1107 w1109 w1110 w1111 w1112]
    tunnel: [w1102 w1103 w1104 w1109 w1110 w1111 w1112] -> w9
    frame "invalid app kind", Default {
    }
    frame "Development System" {
    }
    frame "Run Time System" {
      # "Close FP when ran as an .exe..."
      n392 = control-ref of="This VI"() -> (w1108:refnum<vi>)
      n393 = invoke class="VI" method="FP.Close"(reference=w1108, error in=w1107) -> (reference out=w1105:refnum<vi>, error out=w1106:errorcluster)  [unwired: 1 in, 1 out]
      n394 = Close Reference(reference=w1105, error in (no error)=w1106) -> (error out=w1104:errorcluster)
    }
    frame "Student Edition" {
    }
    frame "Embedded LabVIEW" {
    }
    frame "Evaluation" {
    }
    frame "Custom" {
    }
  }
  n395 = call <vilib>:"Simple Error Handler.vi"("type of dialog (OK msg:1)"=w8, "error in (no error)"=w9) -> ("error out"=→"error out":errorcluster)  [unwired: 3 in, 4 out]
